vi "Live Capture Functional Stack.9.64bit.vi"() -> ()   [LabVIEW 2014]
uses:
  subvis/Stack Track.ctl
  subvis/Stack_State.ctl
  CameraControlTypeDef.ctl
  Desktop/camtiff/ctiff.llb/__CTIFFNewFileAndStyleUINT16.vi
  Desktop/camtiff/ctiff.llb/__CTIFFAddNewPageUINT16.vi
panel:
  in  "Preview":bool
  in  "Capture Mode":bool
  out "Record Ready":bool
  in  "Stacks":dbl=1.0
  in  "Time Lapse":bool
  out "Stack Frames":i32=100
  in  "Stack Frames":i32=100
  in  "Temp":path=path "C:/temp.tmp"
  in  "Frames":i32=100
  in  "HardDisk Record":bool
  in  "Internal Line Interval":dbl
  in  "Slit Width / Lines":sgl=150.0
  in  "Camera Readout Mode":u16(ring)=12 items=["Full Frame"=1, "Slit Scanning"=12]
  in  "Readout Direction":sgl(ring)=1.0 items=["Forward"=1, "Backward"=2]
  in  "Trigger Mode":sgl(ring)=1.0 items=["Normal"=1, "Start "=6]
  in  "Trigger Source":sgl(ring)=2.0 items=["Internal"=1, "External"=2]
  out "State":T1=enum."Start Sequence"
  out "Image":u16[][](graph)
  out "Saving":bool
  in  "AutoIncrement":bool=TRUE
  in  "Path":path=path "C:/Users/spim/Desktop/Craig Cap/temp/a.tiff"
  in  "Frames":i32=100
  out "Frame Index":i32
  out "error out":errorcluster
  in  "stop":bool
  in  "Ram Record":bool
  out "Total Frames":i32
  out "Elapsed Time":u32
  out "Software FPS":dbl
  out "Camera FPS":dbl
  in  "H Offset":i32 min=0 max=0 step=4
  in  "H Width":i32 min=4 max=2048 step=4
  out "SMD":dbl
  out "SHO":i32
  in  "V Offset":i32 min=0 max=0 step=4
  in  "V Width":i32 min=4 max=2048 step=4
  in  "Binning":u16(ring) items=["1x1"=1, "2x2"=2, "4x4"=4]
  out "SHW":i32
  out "SVO":i32
  out "SVW":i32
  in  "Scan Mode":dbl min=1.0 max=2.0 step=1.0
  in  "Exposure":dbl min=0.0010036691729323308 max=10.000004210526315 step=1e-08
  out "EXP":dbl
  out "Camera Model":string
  out "Camera Version":string
  out "Camera Serial":string
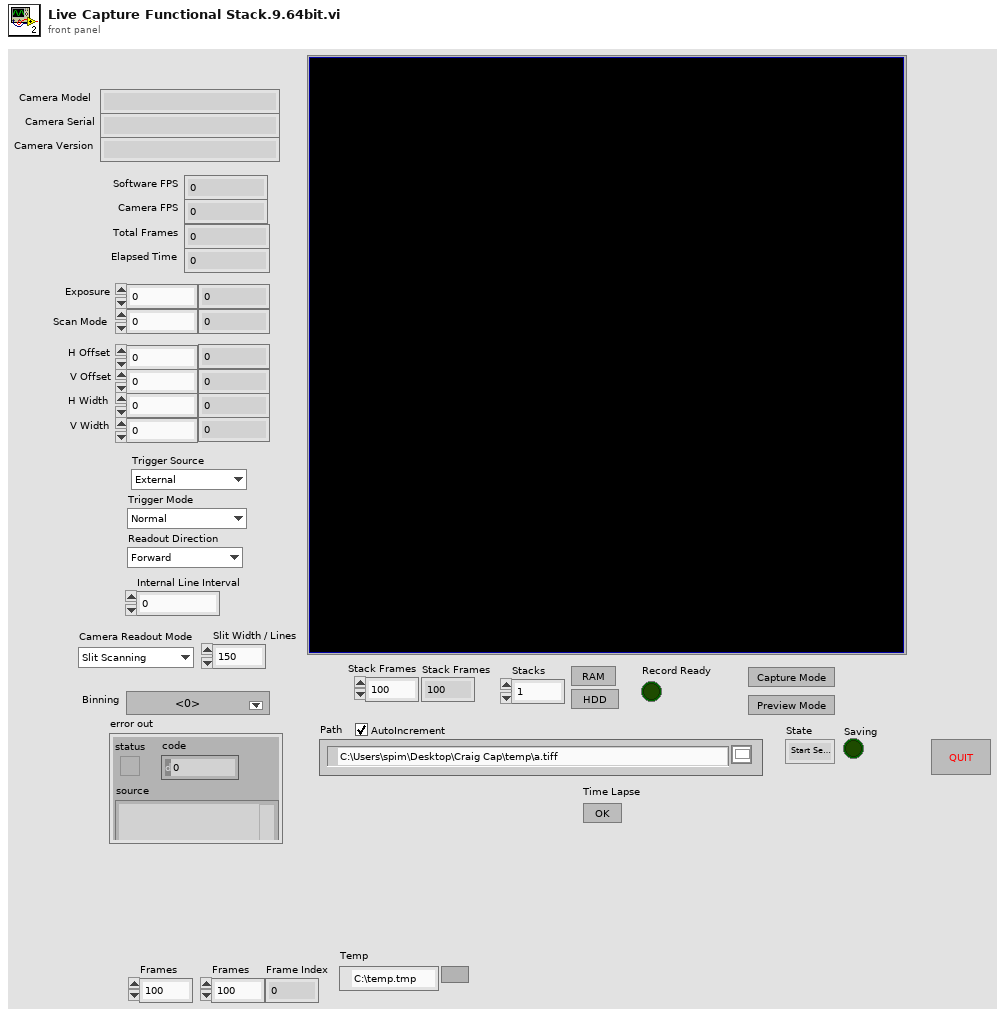
[diagram p1: front panel]
types:
  T1 = typedef "Stack Track.ctl" = enum16{"Idle", "Start Sequence", "Read Disk", "STOP", "Collecting", "End"}
  T2 = typedef "CameraControlTypeDef.ctl" = enum16{"IntervalLineInt", "Ram Record", "HardDisk Record", "Disengage Update", "Update", "Idle", "ROI", "Binning", "Scan Mode", "Trigger Mode", "Readout Mode", "Readout Direction", "Preview"}
  T3 = typedef "Stack_State.ctl" = cluster{"State":T1, "Stack Number":i32, "Image":u16[][]}
  T4 = enum8{"Enabled", "Disabled", "Disabled and Grayed Out"}
  T5 = cluster{"Model":string, "Camera ID":string, "Firmware":string}
  T6 = cluster{"Value":i32, "Minimum":i32, "Maximum":i32, "Increment":i32}
  T7 = cluster{"height":u32, "width":u32, "datatype":u32}
  T8 = cluster{"H Offset":i32, "V Offset":i32, "H Width":i32, "V Width":i32}
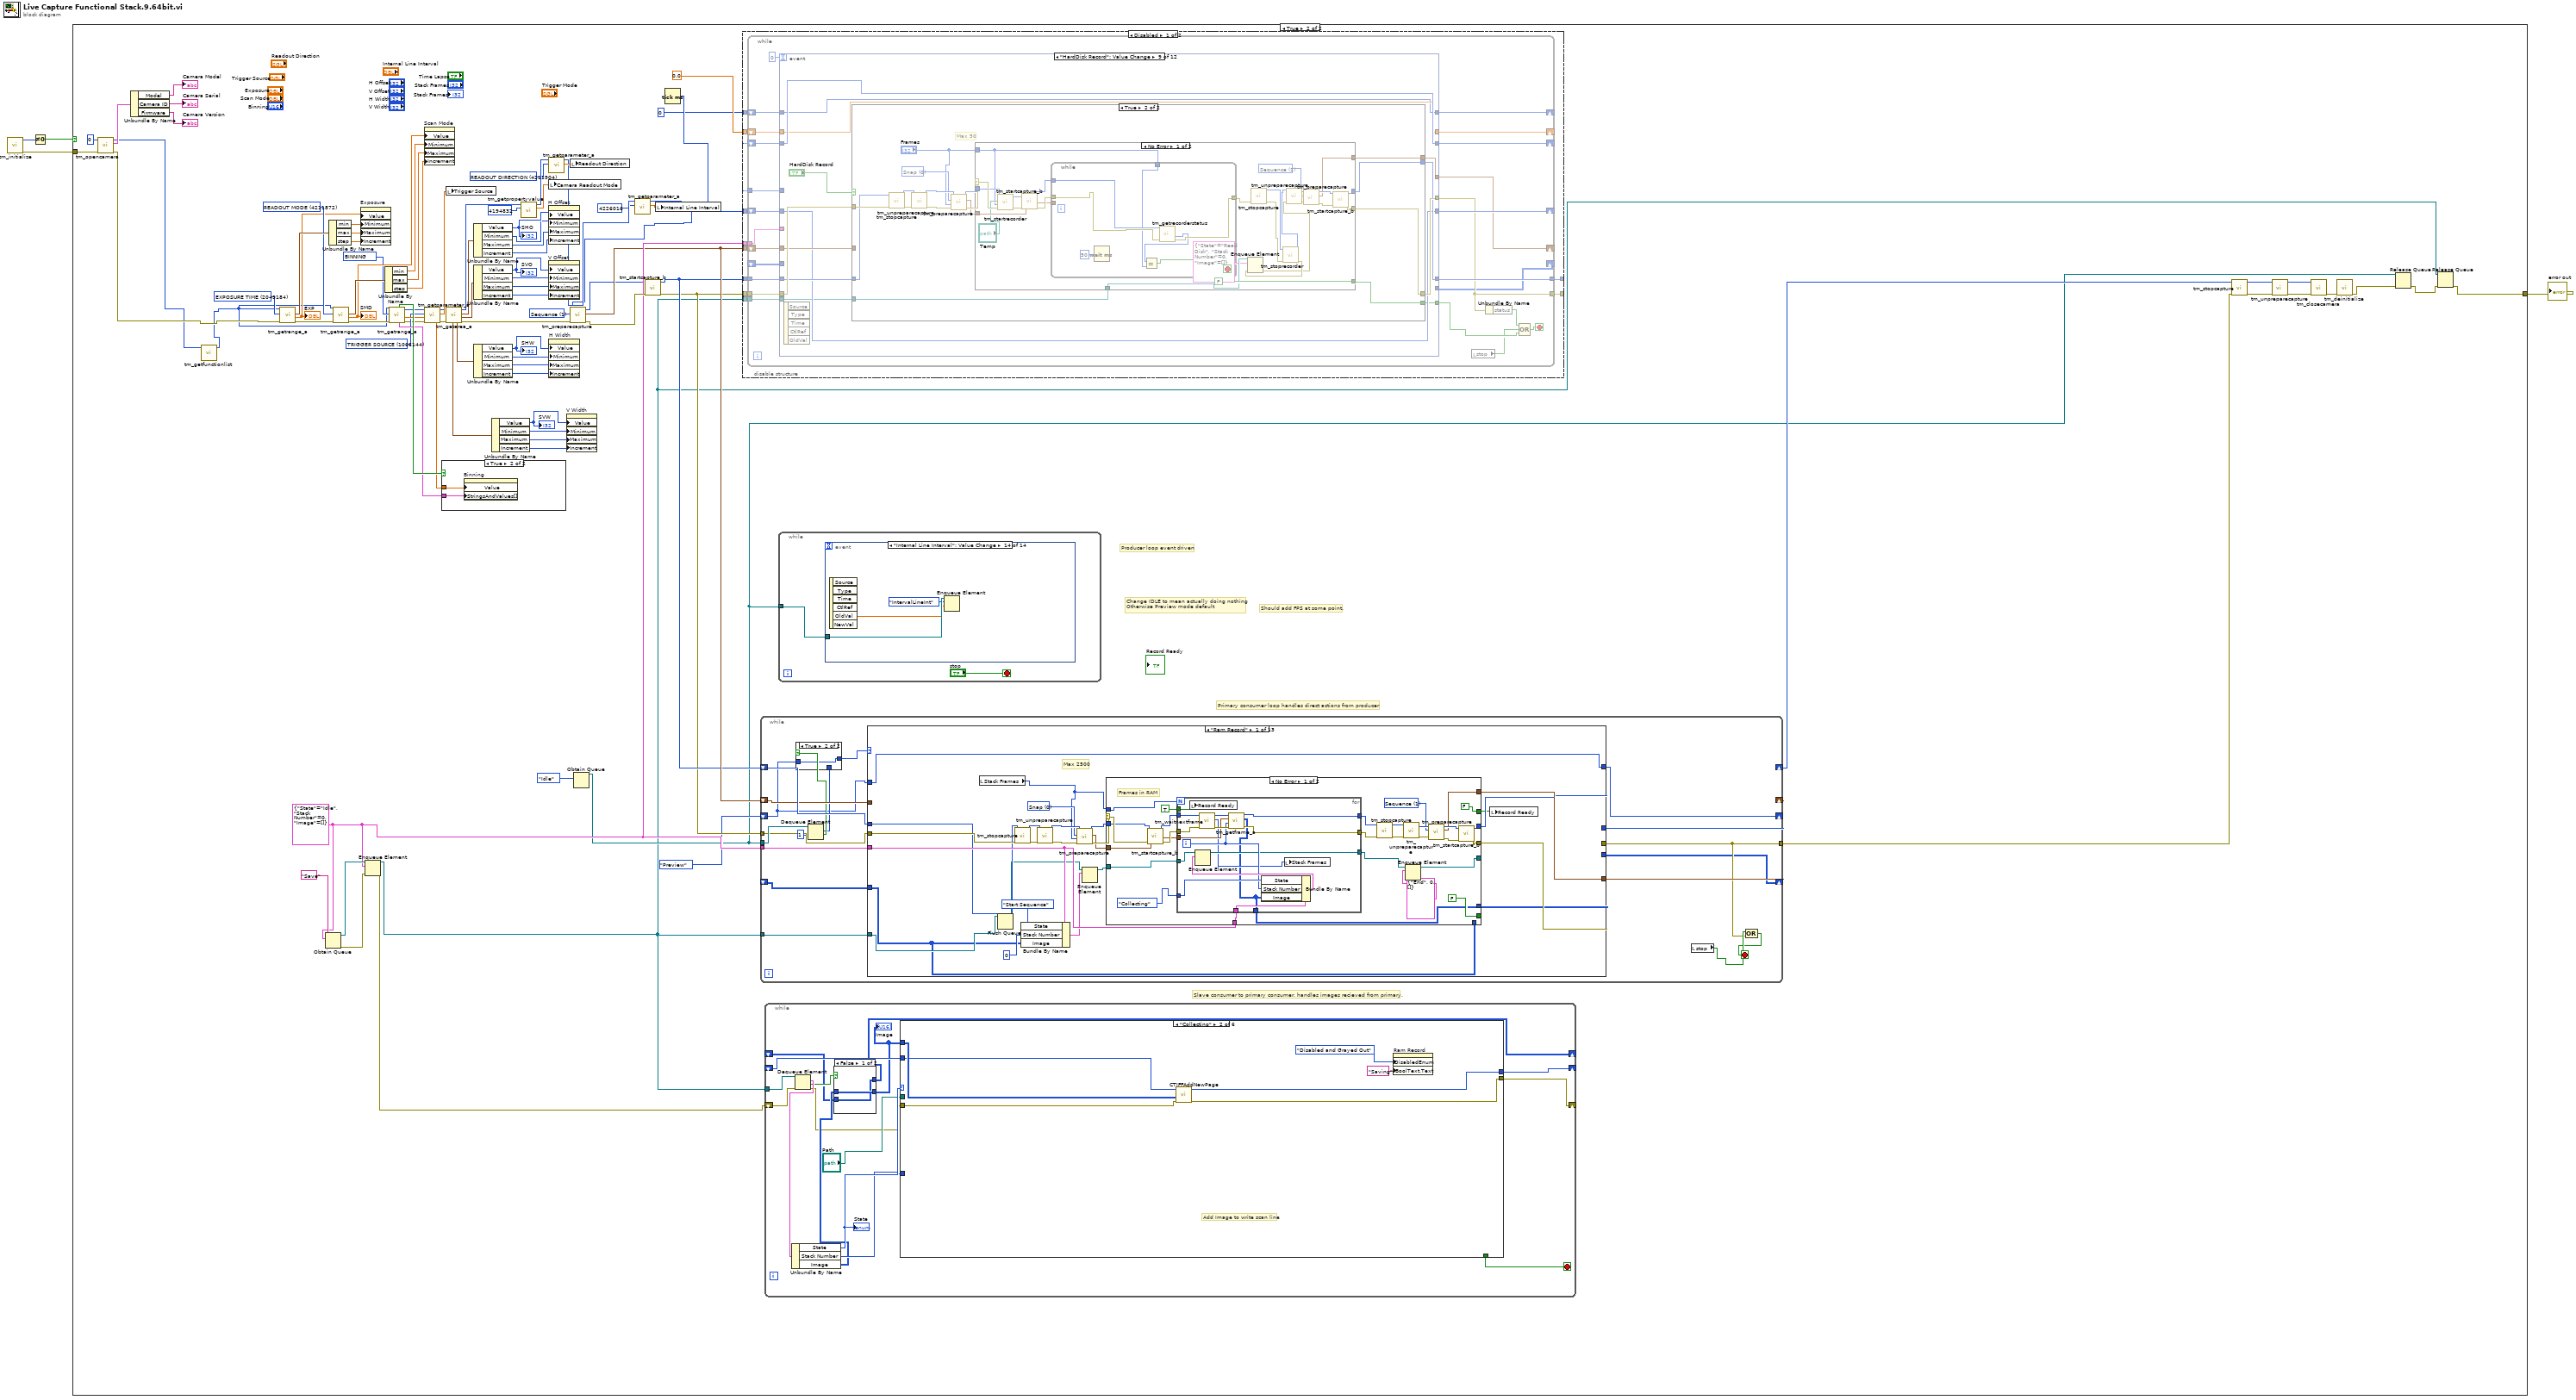
[diagram p0: block diagram]
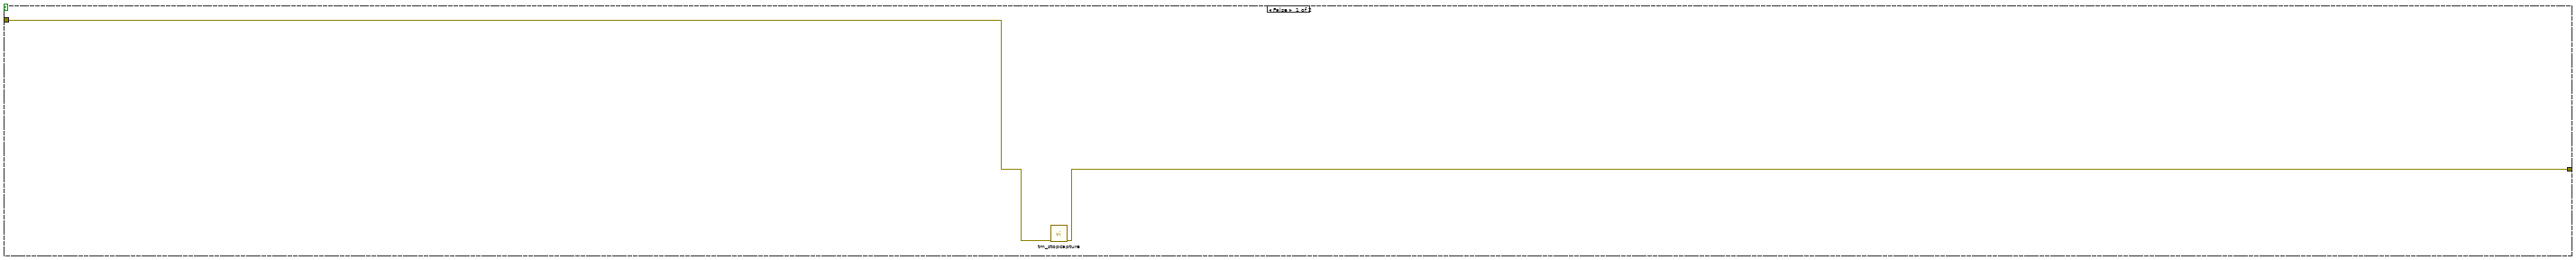
[diagram p2: hidden frame]
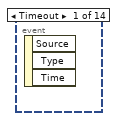
[diagram p3: hidden frame]
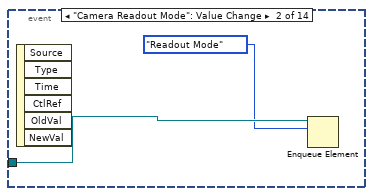
[diagram p4: hidden frame]
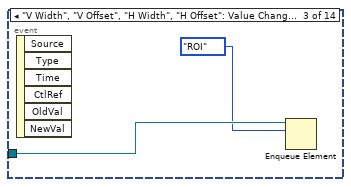
[diagram p5: hidden frame]
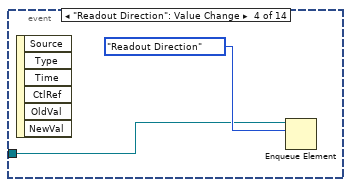
[diagram p6: hidden frame]
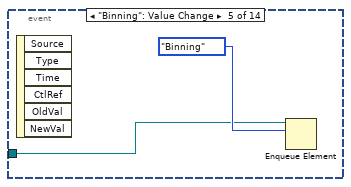
[diagram p7: hidden frame]
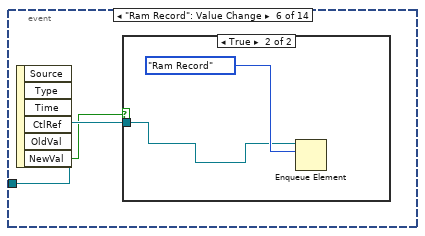
[diagram p8: hidden frame]
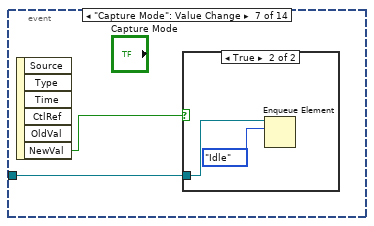
[diagram p10: hidden frame]
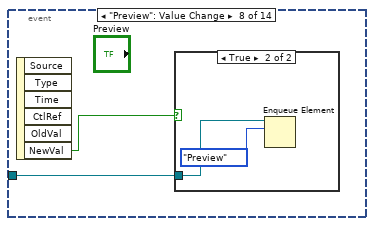
[diagram p12: hidden frame]
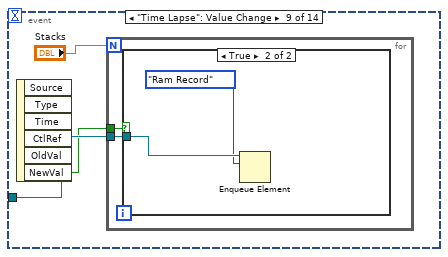
[diagram p14: hidden frame]
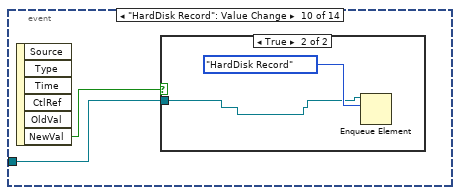
[diagram p16: hidden frame]
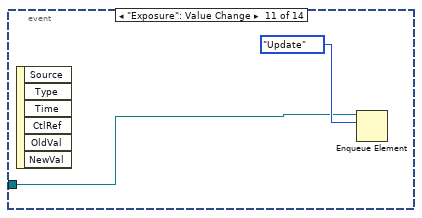
[diagram p18: hidden frame]
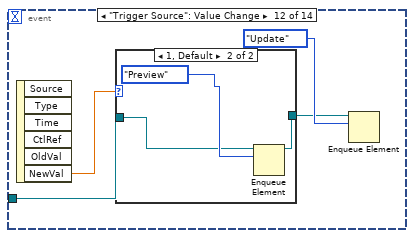
[diagram p19: hidden frame]
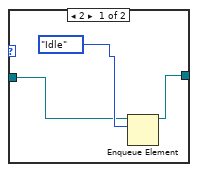
[diagram p20: hidden frame]
diagram:
  n1 = call <userlib>:"tm_initialize.vi"() -> ("error out"=w2:errorcluster, "Number Of Cameras"=w1:u32)  [unwired: 8 in, 2 out]
  n2 = Not Equal To 0?(x=w1) -> (x != 0?=w4:bool)
  n3 = case shown="True" w4 {
    tunnel: [w5 w15] -> w3
    tunnel: w2 -> [w6 w98]
    frame False {
      n4 = call <userlib>:"tm_stopcapture.vi"("error in (no error)"=w6) -> ("error out"=w5:errorcluster)  [unwired: 9 in, 1 out]
    }
    frame True {
      w33 = u32 4211904 items=["SENSOR MODE"=4212128, "CCD MODE"=4212384, "READOUT MODE"=4211872, "ACTIVE VIEW INDEX"=4343136, "BITS PER CHANNEL"=4342976, "IMAGE PIXEL TYPE"=4343296, "BINNING"=4215968, "EXPOSURE TIME"=2049184, "CONTRAST GAIN"=3163312, "CONTRAST OFFSET"=3163328, "LIGHT MODE"=2114720, "SENSITIVITY"=2114992, "PHOTON IMAGING MODE"=2115200, "HIGH DYNAMIC RANGE MODE"=3163360, "WHITE BALANCE"=3163568, "TEMPERATURE"=2115232, "TEMPERATURE TARGET"=2115264, "SENSOR COOLER FAN"=2115296, "LINEBUNDLE HEIGHT"=4212192, "MECHANICAL SHUTTER"=2115488, "BACK FOCUS POSITION"=8422304, "TRIGGER CONNECTOR"=1066432, "TRIGGER SOURCE"=1066144, "OUTPUT TRIGGER SOURCE"=1852576, "TRIGGER GLOBAL EXPOSURE"=2049680, "FIRST TRIGGER BEHAVIOR"=2049696, "CHANNEL SYNC"=1852352, "READOUT DIRECTION"=4211904, "PRE HSYNC COUNT"=1852704] ("Parameter")
      w42 = u32 1066144 items=["SENSOR MODE"=4212128, "CCD MODE"=4212384, "READOUT MODE"=4211872, "ACTIVE VIEW INDEX"=4343136, "BITS PER CHANNEL"=4342976, "IMAGE PIXEL TYPE"=4343296, "BINNING"=4215968, "EXPOSURE TIME"=2049184, "CONTRAST GAIN"=3163312, "CONTRAST OFFSET"=3163328, "LIGHT MODE"=2114720, "SENSITIVITY"=2114992, "PHOTON IMAGING MODE"=2115200, "HIGH DYNAMIC RANGE MODE"=3163360, "WHITE BALANCE"=3163568, "TEMPERATURE"=2115232, "TEMPERATURE TARGET"=2115264, "SENSOR COOLER FAN"=2115296, "LINEBUNDLE HEIGHT"=4212192, "MECHANICAL SHUTTER"=2115488, "BACK FOCUS POSITION"=8422304, "TRIGGER CONNECTOR"=1066432, "TRIGGER SOURCE"=1066144, "OUTPUT TRIGGER SOURCE"=1852576, "TRIGGER GLOBAL EXPOSURE"=2049680, "FIRST TRIGGER BEHAVIOR"=2049696, "CHANNEL SYNC"=1852352, "READOUT DIRECTION"=4211904, "PRE HSYNC COUNT"=1852704] ("Parameter")
      w28 = T3 {"State"=enum."Idle", "Stack Number"=0, "Image"=[]} ("input cluster")
      w47 = u32 2049184 items=["BINNING"=4215968, "BITS PER CHANNEL"=4342976, "ACTIVE VIEW INDEX"=4343136, "CCD MODE"=4212384, "SENSOR MODE"=4212128, "READOUT MODE"=4211872, "EXPOSURE TIME"=2049184, "CONTRAST GAIN"=3163312, "CONTRAST OFFSET"=3163328, "LIGHT MODE"=2114720, "SENSITIVITY"=2114992, "WHITE BALANCE"=3163568, "PHOTON IMAGING MODE"=2115200, "HIGH DYNAMIC RANGE MODE"=3163360, "TRIGGER SOURCE"=1066144, "TRIGGER ACTIVE"=1066160, "TRIGGER MODE"=1066400, "TRIGGER POLARITY"=1066416, "TRIGGER GLOBAL EXPOSURE"=2049680, "FIRST TRIGGER BEHAVIOR"=2049696, "TRIGGER TIMES"=1066448, "OUTPUT TRIGGER POLARITY"=1852592, "OUTPUT TRIGGER DELAY"=1852624, "OUTPUT TRIGGER PERIOD"=1852640, "TEMPERATURE"=2115232, "TEMPERATURE TARGET"=2115264, "SENSOR COOLER FAN"=2115296, "MECHANICAL SHUTTER"=2115488, "BACK FOCUS POSITION"=8422304, "FRAMEBUNDLE MODE"=4346784, "FRAMEBUNDLE NUMBER"=4346800, "LINEBUNDLE HEIGHT"=4212192, "TRIGGER CONNECTOR"=1066432, "IMAGE PIXEL TYPE"=4343296, "OUTPUT TRIGGER KIND"=1852656, "READOUT DIRECTION"=4211904, "CHANNEL SYNC"=1852352] ("Parameter")
      w48 = u32 4211872 items=["BINNING"=4215968, "BITS PER CHANNEL"=4342976, "ACTIVE VIEW INDEX"=4343136, "CCD MODE"=4212384, "SENSOR MODE"=4212128, "READOUT MODE"=4211872, "EXPOSURE TIME"=2049184, "CONTRAST GAIN"=3163312, "CONTRAST OFFSET"=3163328, "LIGHT MODE"=2114720, "SENSITIVITY"=2114992, "WHITE BALANCE"=3163568, "PHOTON IMAGING MODE"=2115200, "HIGH DYNAMIC RANGE MODE"=3163360, "TRIGGER SOURCE"=1066144, "TRIGGER ACTIVE"=1066160, "TRIGGER MODE"=1066400, "TRIGGER POLARITY"=1066416, "TRIGGER GLOBAL EXPOSURE"=2049680, "FIRST TRIGGER BEHAVIOR"=2049696, "TRIGGER TIMES"=1066448, "OUTPUT TRIGGER POLARITY"=1852592, "OUTPUT TRIGGER DELAY"=1852624, "OUTPUT TRIGGER PERIOD"=1852640, "TEMPERATURE"=2115232, "TEMPERATURE TARGET"=2115264, "SENSOR COOLER FAN"=2115296, "MECHANICAL SHUTTER"=2115488, "BACK FOCUS POSITION"=8422304, "FRAMEBUNDLE MODE"=4346784, "FRAMEBUNDLE NUMBER"=4346800, "LINEBUNDLE HEIGHT"=4212192, "TRIGGER CONNECTOR"=1066432, "IMAGE PIXEL TYPE"=4343296, "OUTPUT TRIGGER KIND"=1852656, "READOUT DIRECTION"=4211904, "CHANNEL SYNC"=1852352] ("Parameter")
      w49 = u32 4215968 items=["BINNING"=4215968, "BITS PER CHANNEL"=4342976, "ACTIVE VIEW INDEX"=4343136, "CCD MODE"=4212384, "SENSOR MODE"=4212128, "READOUT MODE"=4211872, "EXPOSURE TIME"=2049184, "CONTRAST GAIN"=3163312, "CONTRAST OFFSET"=3163328, "LIGHT MODE"=2114720, "SENSITIVITY"=2114992, "WHITE BALANCE"=3163568, "PHOTON IMAGING MODE"=2115200, "HIGH DYNAMIC RANGE MODE"=3163360, "TRIGGER SOURCE"=1066144, "TRIGGER ACTIVE"=1066160, "TRIGGER MODE"=1066400, "TRIGGER POLARITY"=1066416, "TRIGGER GLOBAL EXPOSURE"=2049680, "FIRST TRIGGER BEHAVIOR"=2049696, "TRIGGER TIMES"=1066448, "OUTPUT TRIGGER POLARITY"=1852592, "OUTPUT TRIGGER DELAY"=1852624, "OUTPUT TRIGGER PERIOD"=1852640, "TEMPERATURE"=2115232, "TEMPERATURE TARGET"=2115264, "SENSOR COOLER FAN"=2115296, "MECHANICAL SHUTTER"=2115488, "BACK FOCUS POSITION"=8422304, "FRAMEBUNDLE MODE"=4346784, "FRAMEBUNDLE NUMBER"=4346800, "LINEBUNDLE HEIGHT"=4212192, "TRIGGER CONNECTOR"=1066432, "IMAGE PIXEL TYPE"=4343296, "OUTPUT TRIGGER KIND"=1852656, "READOUT DIRECTION"=4211904, "CHANNEL SYNC"=1852352] ("Parameter")
      w94 = 1 items=["Snap", "Sequence"] ("Capture mode")
      # "Change IDLE to mean actually doing nothing\nOtherwise Preview mode default"
      # "Slave consumer to primary consumer, handles images recieved from primary."
      # "Primary consumer loop handles direct actions from producer"
      # "Producer loop event driven"
      # "Should add FPS at some point."
      n5 = call <userlib>:"tm_opencamera.vi"("error in (no error)"=w98, "Camera Index"=u32 0) -> ("error out"=w29:errorcluster, "Camera Details"=w61:T5, "Handle out"=w13:u32)  [unwired: 7 in]
      n6 = Unbundle By Name(w61) -> ("Model"=→"Camera Model":string, "Camera ID"=→"Camera Serial":string, "Firmware"=→"Camera Version":string)
      n7 = call <userlib>:"tm_getfunctionlist.vi"("Handle in"=w13) -> ("Handle out"=w12:u32)  [unwired: 8 in, 2 out]
      n8 = call <userlib>:"tm_getrange_a.vi"("error in (no error)"=w29, "Parameter"=w47, "Handle in"=w12) -> ("error out"=w56:errorcluster, "default"=w45:dbl, "Range"=w57:cluster{"min":dbl, "max":dbl, "step":dbl})  [unwired: 2 in, 4 out]
      "EXP" <- w45
      n9 = Obtain Queue(name (unnamed)="Save", element data type=w28) -> (queue out=w31:refnum<queue>, error out=w10:errorcluster)  [unwired: 3 in, 1 out]
      n10 = Unbundle By Name(w57) -> ("min"=w92:dbl, "max"=w91:dbl, "step"=w90:dbl)
      n11 = call <userlib>:"tm_getrange_a.vi"("error in (no error)"=w56, "Parameter"=w48, "Handle in"=w12) -> ("error out"=w53:errorcluster, "default"=w54:dbl, "Range"=w55:cluster{"min":dbl, "max":dbl, "step":dbl})  [unwired: 2 in, 4 out]
      "SMD" <- w54
      n12 = property on="Exposure" class="DigNum (strict)"("Value"=w45, "Minimum"=w92, "Maximum"=w91, "Increment"=w90) -> ()  [unwired: 2 in, 2 out]
      n13 = Enqueue Element(queue=w31, element=w28, error in (no error)=w10) -> (queue out=w14:refnum<queue>, error out=w9:errorcluster)  [unwired: 1 in, 1 out]
      n14 = Unbundle By Name(w55) -> ("min"=w89:dbl, "max"=w88:dbl, "step"=w87:dbl)
      n15 = call <userlib>:"tm_getrange_a.vi"("error in (no error)"=w53, "Parameter"=w49, "Handle in"=w12) -> ("error out"=w39:errorcluster, "default"=w51:dbl, "Handle out"=w41:u32, "Value Names"=w50:cluster{"Name":string, "Value":dbl}[], "Writable"=w52:bool)  [unwired: 2 in, 2 out]
      n16 = property on="Scan Mode" class="DigNum (strict)"("Value"=w54, "Minimum"=w89, "Maximum"=w88, "Increment"=w87) -> ()  [unwired: 2 in, 2 out]
      n17 = call <userlib>:"tm_getparameter_a.vi"("error in (no error)"=w39, "Parameter"=w42, "Handle in"=w41) -> ("error out"=w38:errorcluster, "Value out"=w43:dbl, "Handle out"=w40:u32)  [unwired: 6 in]
      n18 = case shown="True" w52 {
        tunnel: w50 -> [_ w1177]
        tunnel: w51 -> [_ w1176]
        frame False {
        }
        frame True {
          n19 = property on="Binning" class="Ring (strict)"("Value"=w1176, "StringsAndValues[]"=w1177) -> ()  [unwired: 2 in, 2 out]
        }
      }
      n20 = local write "Trigger Source"(w43) -> ()
      n21 = call <userlib>:"tm_getarea_a.vi"("error in (no error)"=w38, "Handle in"=w40) -> ("error out"=w44:errorcluster, "V Offset"=w86:T6, "H Offset"=w67:T6, "Handle out"=w35:u32, "H Width"=w85:T6, "V Width"=w84:T6)  [unwired: 4 in]
      n22 = Unbundle By Name(w67) -> ("Value"=w66:i32, "Minimum"=w65:i32, "Maximum"=w64:i32, "Increment"=w63:i32)
      "SHO" <- w66
      n23 = Unbundle By Name(w86) -> ("Value"=w74:i32, "Minimum"=w83:i32, "Maximum"=w82:i32, "Increment"=w81:i32)
      "SVO" <- w74
      n24 = Unbundle By Name(w85) -> ("Value"=w73:i32, "Minimum"=w80:i32, "Maximum"=w79:i32, "Increment"=w78:i32)
      "SHW" <- w73
      n25 = Unbundle By Name(w84) -> ("Value"=w72:i32, "Minimum"=w77:i32, "Maximum"=w76:i32, "Increment"=w75:i32)
      "SVW" <- w72
      n26 = call <userlib>:"tm_getpropertyvalue.vi"("Property ID"=u32 4194832, "Handle in"=w35) -> ("Value in"=w36:sgl, "Handle out"=w34:u32)  [unwired: 7 in, 1 out]
      n27 = call <userlib>:"tm_getparameter_a.vi"("Parameter"=w33, "Handle in"=w34) -> ("Value out"=w32:dbl, "Handle out"=w19:u32)  [unwired: 7 in, 1 out]
      n28 = local write "Camera Readout Mode"(w36) -> ()
      n29 = property on="H Offset" class="DigNum (strict)"("Value"=w66, "Minimum"=w65, "Maximum"=w64, "Increment"=w63) -> ()  [unwired: 2 in, 2 out]
      n30 = property on="V Offset" class="DigNum (strict)"("Value"=w74, "Minimum"=w83, "Maximum"=w82, "Increment"=w81) -> ()  [unwired: 2 in, 2 out]
      n31 = property on="H Width" class="DigNum (strict)"("Value"=w73, "Minimum"=w80, "Maximum"=w79, "Increment"=w78) -> ()  [unwired: 2 in, 2 out]
      n32 = property on="V Width" class="DigNum (strict)"("Value"=w72, "Minimum"=w77, "Maximum"=w76, "Increment"=w75) -> ()  [unwired: 2 in, 2 out]
      n33 = local write "Readout Direction"(w32) -> ()
      n34 = Obtain Queue(element data type=CameraControlTypeDef."Idle" ("Enum")) -> (queue out=w17:refnum<queue>)  [unwired: 4 in, 2 out]
      n35 = call <userlib>:"tm_getparameter_a.vi"("Parameter"=4226016, "Handle in"=w19) -> ("Value out"=w7:dbl, "Handle out"=w8:u32)  [unwired: 7 in, 1 out]
      n36 = call <userlib>:"tm_preparecapture.vi"("error in (no error)"=w44, "Capture mode"=w94, "Handle in"=w8) -> ("error out"=w30:errorcluster, "Buffer Info"=w27:T7, "Handle out"=w20:u32)  [unwired: 5 in, 1 out]
      n37 = call <userlib>:"tm_startcapture_b.vi"("error in (no error)"=w30, "Handle in"=w20) -> ("error out"=w25:errorcluster, "Handle out"=w26:u32)  [unwired: 8 in]
      n38 = local write "Internal Line Interval"(w7) -> ()
      n39 = Tick Count (ms)() -> (millisecond timer value=w93:u32)
      n40 = disable-structure shown="Disabled" {
        disable-tunnel: 0.0 -> [w592 _]
        disable-tunnel: w93 -> [w591 _]
        disable-tunnel: 0 -> [w590 _]
        disable-tunnel: [w589 _] -> _
        disable-tunnel: [w588 _] -> _
        disable-tunnel: w28 -> [w587 _]
        disable-tunnel: w27 -> [w586 _]
        disable-tunnel: w26 -> [w585 _]
        disable-tunnel: w25 -> [w584 _]
        disable-tunnel: w14 -> [w583 _]
        frame Disabled {
          n41 = while {
            tunnel: w584 -> [w606]
            tunnel: [w604] -> w588
            tunnel: [w603] -> w589
            shift-right: [w613] -> _
            shift-left: w591 -> [w611]
            shift-right: [w614] -> _
            shift-left: w592 -> [w612]
            shift-right: [w605] -> _
            shift-left: w591 -> [w609]
            tunnel: w585 -> [w607]
            tunnel: w591 -> [w610]
            shift-right: [w602] -> _
            shift-left: w586 -> [w608]
            shift-right: [w600] -> _
            shift-left: w590 -> [w601]
            tunnel: w583 -> [w599]
            shift-right: [w597] -> _
            shift-left: _ -> [w596]
            tunnel: w587 -> [w595]
            stop <- w615 stop-if-true
            n42 = event shown="[8] \"HardDisk Record\": Value Change" {
              selector: _ -> [_ _ _ _ _ _ _ _ _ _ _ _]
              dyn-events: _ -> [_ _ _ _ _ _ _ _ _ _ _ _]
              timeout: 0 -> [_ _ _ _ _ _ _ _ _ _ _ _]
              tunnel: [w626 w695 w709 w722 w741 w761 w783 w811 w908 w1002 w1038 w1083] -> w614
              tunnel: [w625 w696 w710 w723 w742 w762 w784 w812 w909 w1003 w1039 w1084] -> w613
              tunnel: w612 -> [w637 w695 w709 w722 w741 w761 w783 w811 w908 w1002 w1038 w1083]
              tunnel: w611 -> [w628 w696 w710 w723 w742 w762 w784 w812 w909 w1003 w1039 w1084]
              tunnel: w610 -> [w633 _ _ _ _ _ _ _ _ _ _ _]
              tunnel: w609 -> [w638 w697 w711 w724 w743 w763 w785 w807 w904 w1004 w1046 w1091]
              tunnel: w608 -> [w632 w694 w708 w721 _ w760 _ w808 w905 _ _ _]
              tunnel: w607 -> [w640 w690 w703 w717 w736 w754 w776 w815 w912 w999 w1015 w1053]
              tunnel: w606 -> [w639 w692 w699 w718 w735 w757 w775 w816 w913 w998 w1014 w1052]
              tunnel: [w636 w697 w711 w724 w743 w763 w785 w807 w904 w1004 w1046 w1091] -> w605
              tunnel: [w635 w687 w706 w714 w727 w747 w766 w813 w910 w993 w1041 w1086] -> w604
              tunnel: [w634 w686 w705 w713 w726 w746 w764 w814 w911 w994 w1042 w1087] -> w603
              tunnel: [w631 w694 w708 w721 w730 w760 w771 w809 w906 w992 w1040 w1085] -> w602
              tunnel: w601 -> [w623 w693 w707 w720 w740 w759 w782 w810 w907 w991 w1011 w1047]
              tunnel: [w622 w693 w707 w720 w740 w759 w782 w810 w907 w991 w1011 w1047] -> w600
              tunnel: w599 -> [w617 _ _ _ _ _ _ w806 w903 _ _ _]
              tunnel: [_ _ _ _ _ _ _ w805 w902 _ _ _] -> w598
              tunnel: w595 -> [w620 _ _ _ _ _ _ w803 _ _ _ _]
              tunnel: [w619 _ _ _ _ _ _ _ _ _ _ _] -> w597
              tunnel: w596 -> [w618 _ _ _ _ _ _ w804 _ _ _ _]
              event Timeout {
                n43 = event-data() -> ()  [unwired: 1 in, 2 out]
                n44 = call <userlib>:"tm_waitnextframe.vi"("error in (no error)"=w639, "Handle in"=w640) -> ("error out"=w643:errorcluster, "Frame Count"=w624:i32, "Frame Index"=w642:i32, "Handle out"=w644:u32)  [unwired: 6 in]
                "Total Frames" <- w624
                n45 = Tick Count (ms)() -> (millisecond timer value=w630:u32)
                n46 = Increment(x=w637) -> (x+1=w627:dbl)
                n47 = Subtract(x=w630, y=w633) -> (x-y=→"Elapsed Time":u32)
                n48 = Add(x=w628, y=u32 1000) -> (x+y=w648:u32)
                n49 = Less Or Equal?(x=w648, y=w630) -> (x <= y?=w629:bool)
                n50 = Add(x=w638, y=u32 50) -> (x+y=w646:u32)
                n51 = Less Or Equal?(x=w646, y=w630) -> (x <= y?=w621:bool)
                n52 = case shown="True" w629 {
                  tunnel: w628 -> [w651 w660]
                  tunnel: [w651 w657] -> w625
                  tunnel: w627 -> [w650 w663]
                  tunnel: w630 -> [_ w657]
                  tunnel: [w650 0.0] -> w626
                  tunnel: w624 -> [_ w652]
                  tunnel: w623 -> [w649 w655]
                  tunnel: [w649 w652] -> w622
                  frame False {
                  }
                  frame True {
                    n53 = Subtract(x=w657, y=w660) -> (x-y=w659:u32)
                    n54 = Subtract(x=w652, y=w655) -> (x-y=w653:i32)
                    n55 = To Double Precision Float(number=w659) -> (double precision float=w665:dbl)
                    n56 = Divide(x=w665, y=1000.0) -> (x/y=w656:dbl)
                    n57 = To Double Precision Float(number=w653) -> (double precision float=w654:dbl)
                    n58 = Divide(x=w654, y=w656) -> (x/y=→"Camera FPS":dbl)
                    n59 = Divide(x=w663, y=w656) -> (x/y=→"Software FPS":dbl)
                  }
                }
                n60 = case shown="True" w621 {
                  tunnel: w638 -> [w670 _]
                  tunnel: w630 -> [_ w683]
                  tunnel: [w670 w683] -> w636
                  tunnel: w644 -> [w669 w682]
                  tunnel: w632 -> [w667 w677]
                  tunnel: w643 -> [w668 w681]
                  tunnel: [w669 w680] -> w635
                  tunnel: [w668 w679] -> w634
                  tunnel: w642 -> [_ w678]
                  tunnel: [w667 w677] -> w631
                  tunnel: w617 -> [_ w676]
                  tunnel: w620 -> [_ w672]
                  tunnel: [w666 w671] -> w619
                  tunnel: w618 -> [w666 _]
                  frame False {
                  }
                  frame True {
                    n61 = call <userlib>:"tm_getframe_a.vi"("error in (no error)"=w681, "Frame Index"=w678, "Buffer Info"=w677, "Handle in"=w682) -> ("error out"=w679:errorcluster, "Data 16"=w671:u16[][], "Handle out"=w680:u32)  [unwired: 3 in, 2 out]
                    n62 = Bundle By Name(cluster=w672, "State"=Stack_Track."Idle", "Stack Number"=0, "Image"=w671) -> (w673:T3)
                    n63 = Enqueue Element(queue=w676, element=w673) -> ()  [unwired: 2 in, 3 out]
                  }
                }
              }
              event "Exposure": Value Change {
                w685 = u32 2049184 items=["SENSOR MODE"=4212128, "CCD MODE"=4212384, "READOUT MODE"=4211872, "ACTIVE VIEW INDEX"=4343136, "BITS PER CHANNEL"=4342976, "IMAGE PIXEL TYPE"=4343296, "BINNING"=4215968, "EXPOSURE TIME"=2049184, "CONTRAST GAIN"=3163312, "CONTRAST OFFSET"=3163328, "LIGHT MODE"=2114720, "SENSITIVITY"=2114992, "PHOTON IMAGING MODE"=2115200, "HIGH DYNAMIC RANGE MODE"=3163360, "WHITE BALANCE"=3163568, "TEMPERATURE"=2115232, "TEMPERATURE TARGET"=2115264, "SENSOR COOLER FAN"=2115296, "LINEBUNDLE HEIGHT"=4212192, "MECHANICAL SHUTTER"=2115488, "BACK FOCUS POSITION"=8422304, "TRIGGER CONNECTOR"=1066432, "TRIGGER SOURCE"=1066144, "OUTPUT TRIGGER SOURCE"=1852576, "TRIGGER GLOBAL EXPOSURE"=2049680, "FIRST TRIGGER BEHAVIOR"=2049696, "CHANNEL SYNC"=1852352, "READOUT DIRECTION"=4211904, "PRE HSYNC COUNT"=1852704] ("Parameter")
                n64 = event-data() -> ("NewVal"=w691:dbl)  [unwired: 1 in, 2 out]
                n65 = call <userlib>:"tm_setparameter_a.vi"("error in (no error)"=w692, "Value in"=w691, "Parameter"=w685, "Handle in"=w690) -> ("error out"=w689:errorcluster, "Handle out"=w688:u32)  [unwired: 6 in]
                n66 = call <userlib>:"tm_getparameter_a.vi"("error in (no error)"=w689, "Parameter"=w685, "Handle in"=w688) -> ("error out"=w686:errorcluster, "Value out"=w684:dbl, "Handle out"=w687:u32)  [unwired: 6 in]
                n67 = local write "EXP"(w684) -> ()
              }
              event "Internal Line Interval": Value Change {
                w698 = u32 4191424 items=["SENSOR MODE"=4212128, "CCD MODE"=4212384, "READOUT MODE"=4211872, "ACTIVE VIEW INDEX"=4343136, "BITS PER CHANNEL"=4342976, "IMAGE PIXEL TYPE"=4343296, "BINNING"=4215968, "EXPOSURE TIME"=2049184, "CONTRAST GAIN"=3163312, "CONTRAST OFFSET"=3163328, "LIGHT MODE"=2114720, "SENSITIVITY"=2114992, "PHOTON IMAGING MODE"=2115200, "HIGH DYNAMIC RANGE MODE"=3163360, "WHITE BALANCE"=3163568, "TEMPERATURE"=2115232, "TEMPERATURE TARGET"=2115264, "SENSOR COOLER FAN"=2115296, "LINEBUNDLE HEIGHT"=4212192, "MECHANICAL SHUTTER"=2115488, "BACK FOCUS POSITION"=8422304, "TRIGGER CONNECTOR"=1066432, "TRIGGER SOURCE"=1066144, "OUTPUT TRIGGER SOURCE"=1852576, "TRIGGER GLOBAL EXPOSURE"=2049680, "FIRST TRIGGER BEHAVIOR"=2049696, "CHANNEL SYNC"=1852352, "READOUT DIRECTION"=4211904, "PRE HSYNC COUNT"=1852704, "INTERNAL LINE SPEED"=4191408, "INTERNAL LINE INVERVAL"=4191424] ("Parameter")
                n68 = event-data() -> ("NewVal"=w702:dbl)  [unwired: 1 in, 2 out]
                n69 = call <userlib>:"tm_setparameter_a.vi"("error in (no error)"=w699, "Value in"=w702, "Parameter"=w698, "Handle in"=w703) -> ("error out"=w700:errorcluster, "Handle out"=w701:u32)  [unwired: 6 in]
                n70 = call <userlib>:"tm_getparameter_a.vi"("error in (no error)"=w700, "Parameter"=w698, "Handle in"=w701) -> ("error out"=w705:errorcluster, "Value out"=w704:dbl, "Handle out"=w706:u32)  [unwired: 6 in]
                n71 = local write "Internal Line Interval"(w704) -> ()
              }
              event "Trigger Source": Value Change {
                w719 = u32 1066144 items=["SENSOR MODE"=4212128, "CCD MODE"=4212384, "READOUT MODE"=4211872, "ACTIVE VIEW INDEX"=4343136, "BITS PER CHANNEL"=4342976, "IMAGE PIXEL TYPE"=4343296, "BINNING"=4215968, "EXPOSURE TIME"=2049184, "CONTRAST GAIN"=3163312, "CONTRAST OFFSET"=3163328, "LIGHT MODE"=2114720, "SENSITIVITY"=2114992, "PHOTON IMAGING MODE"=2115200, "HIGH DYNAMIC RANGE MODE"=3163360, "WHITE BALANCE"=3163568, "TEMPERATURE"=2115232, "TEMPERATURE TARGET"=2115264, "SENSOR COOLER FAN"=2115296, "LINEBUNDLE HEIGHT"=4212192, "MECHANICAL SHUTTER"=2115488, "BACK FOCUS POSITION"=8422304, "TRIGGER CONNECTOR"=1066432, "TRIGGER SOURCE"=1066144, "OUTPUT TRIGGER SOURCE"=1852576, "TRIGGER GLOBAL EXPOSURE"=2049680, "FIRST TRIGGER BEHAVIOR"=2049696, "CHANNEL SYNC"=1852352, "READOUT DIRECTION"=4211904, "PRE HSYNC COUNT"=1852704] ("Parameter")
                n72 = event-data() -> ("NewVal"=w712:sgl)  [unwired: 1 in, 3 out]
                n73 = call <userlib>:"tm_setparameter_a.vi"("error in (no error)"=w718, "Value in"=w712, "Parameter"=w719, "Handle in"=w717) -> ("error out"=w716:errorcluster, "Handle out"=w715:u32)  [unwired: 6 in]
                n74 = call <userlib>:"tm_getparameter_a.vi"("error in (no error)"=w716, "Parameter"=w719, "Handle in"=w715) -> ("error out"=w713:errorcluster, "Handle out"=w714:u32)  [unwired: 6 in, 1 out]
              }
              event "Trigger Mode": Value Change {
                w731 = 1 items=["Snap", "Sequence"] ("Capture mode")
                n75 = event-data() -> ("NewVal"=w725:sgl)  [unwired: 1 in, 4 out]
                n76 = call <userlib>:"tm_stopcapture.vi"("error in (no error)"=w735, "Handle in"=w736) -> ("error out"=w738:errorcluster, "Handle out"=w737:u32)  [unwired: 8 in]
                n77 = call <userlib>:"tm_unpreparecapture.vi"("error in (no error)"=w738, "Handle in"=w737) -> ("error out"=w734:errorcluster, "Handle out"=w733:u32)  [unwired: 8 in]
                n78 = call <userlib>:"tm_setpropertyvalue.vi"("error in (no error)"=w734, "Value in"=w725, "Property ID"=u32 1049104, "Handle in"=w733) -> ("error out"=w729:errorcluster, "Handle out"=w732:u32)  [unwired: 6 in]
                n79 = call <userlib>:"tm_preparecapture.vi"("Capture mode"=w731, "Handle in"=w732) -> ("Buffer Info"=w730:T7, "Handle out"=w728:u32)  [unwired: 6 in, 2 out]
                n80 = call <userlib>:"tm_startcapture_b.vi"("error in (no error)"=w729, "Handle in"=w728) -> ("error out"=w726:errorcluster, "Handle out"=w727:u32)  [unwired: 8 in]
              }
              event "Readout Direction": Value Change {
                w752 = 1 items=["Snap", "Sequence"] ("Capture mode")
                w745 = u32 4211904 items=["SENSOR MODE"=4212128, "CCD MODE"=4212384, "READOUT MODE"=4211872, "ACTIVE VIEW INDEX"=4343136, "BITS PER CHANNEL"=4342976, "IMAGE PIXEL TYPE"=4343296, "BINNING"=4215968, "EXPOSURE TIME"=2049184, "CONTRAST GAIN"=3163312, "CONTRAST OFFSET"=3163328, "LIGHT MODE"=2114720, "SENSITIVITY"=2114992, "PHOTON IMAGING MODE"=2115200, "HIGH DYNAMIC RANGE MODE"=3163360, "WHITE BALANCE"=3163568, "TEMPERATURE"=2115232, "TEMPERATURE TARGET"=2115264, "SENSOR COOLER FAN"=2115296, "LINEBUNDLE HEIGHT"=4212192, "MECHANICAL SHUTTER"=2115488, "BACK FOCUS POSITION"=8422304, "TRIGGER CONNECTOR"=1066432, "TRIGGER SOURCE"=1066144, "OUTPUT TRIGGER SOURCE"=1852576, "TRIGGER GLOBAL EXPOSURE"=2049680, "FIRST TRIGGER BEHAVIOR"=2049696, "CHANNEL SYNC"=1852352, "READOUT DIRECTION"=4211904, "PRE HSYNC COUNT"=1852704] ("Parameter")
                n81 = event-data() -> ("NewVal"=w744:sgl)  [unwired: 1 in, 3 out]
                n82 = call <userlib>:"tm_stopcapture.vi"("error in (no error)"=w757, "Handle in"=w754) -> ("error out"=w758:errorcluster, "Handle out"=w753:u32)  [unwired: 8 in]
                n83 = call <userlib>:"tm_unpreparecapture.vi"("error in (no error)"=w758, "Handle in"=w753) -> ("error out"=w756:errorcluster, "Handle out"=w755:u32)  [unwired: 8 in]
                n84 = call <userlib>:"tm_setparameter_a.vi"("error in (no error)"=w756, "Value in"=w744, "Parameter"=w745, "Handle in"=w755) -> ("error out"=w749:errorcluster, "Handle out"=w748:u32)  [unwired: 6 in]
                n85 = call <userlib>:"tm_preparecapture.vi"("error in (no error)"=w749, "Capture mode"=w752, "Handle in"=w748) -> ("error out"=w750:errorcluster, "Handle out"=w751:u32)  [unwired: 5 in, 2 out]
                n86 = call <userlib>:"tm_startcapture_b.vi"("error in (no error)"=w750, "Handle in"=w751) -> ("error out"=w746:errorcluster, "Handle out"=w747:u32)  [unwired: 8 in]
              }
              event "Camera Readout Mode", "Slit Width / Lines": Value Change {
                w769 = 1 items=["Snap", "Sequence"] ("Capture mode")
                n87 = event-data() -> ()  [unwired: 1 in, 4 out]
                n88 = call <userlib>:"tm_stopcapture.vi"("error in (no error)"=w775, "Handle in"=w776) -> ("error out"=w777:errorcluster, "Handle out"=w773:u32)  [unwired: 8 in]
                n89 = call <userlib>:"tm_unpreparecapture.vi"("error in (no error)"=w777, "Handle in"=w773) -> ("error out"=w768:errorcluster, "Handle out"=w774:u32)  [unwired: 8 in]
                n90 = call <userlib>:"tm_setpropertyvalue.vi"("error in (no error)"=w768, "Value in"="Camera Readout Mode", "Property ID"=u32 4194832, "Handle in"=w774) -> ("error out"=w778:errorcluster, "Handle out"=w779:u32)  [unwired: 6 in]
                n91 = case shown="12" "Camera Readout Mode" {
                  tunnel: w779 -> [w790 w797]
                  tunnel: [w789 w792] -> w772
                  tunnel: w778 -> [w787 w802]
                  tunnel: [w786 w802] -> w770
                  frame 1, Default {
                    n92 = local read "Exposure"() -> (w788:dbl)
                    n93 = call <userlib>:"tm_setpropertyvalue.vi"("error in (no error)"=w787, "Value in"=w788, "Property ID"=u32 2031888, "Handle in"=w790) -> ("error out"=w786:errorcluster, "Handle out"=w789:u32)  [unwired: 6 in]
                  }
                  frame 12 {
                    n94 = local read "Exposure"() -> (w801:dbl)
                    n95 = local read "SVW"() -> (w799:i32)
                    n96 = formula code="slitExpos=frameInter*LW/(LinesToReadout\n+10+LW);\nlineInter = slitExpos / LW;"("frameInter"=w801, "LW"="Slit Width / Lines", "LinesToReadout"=w799) -> ("slitExpos"=w793:dbl, "lineInter"=w796:dbl)
                    n97 = call <userlib>:"tm_setpropertyvalue.vi"("Value in"=w796, "Property ID"=u32 4208720, "Handle in"=w797) -> ("Handle out"=w795:u32)  [unwired: 7 in, 1 out]
                    n98 = call <userlib>:"tm_setpropertyvalue.vi"("Value in"=w793, "Property ID"=u32 2031888, "Handle in"=w795) -> ("Handle out"=w792:u32)  [unwired: 7 in, 1 out]
                  }
                }
                n99 = call <userlib>:"tm_preparecapture.vi"("error in (no error)"=w770, "Capture mode"=w769, "Handle in"=w772) -> ("error out"=w765:errorcluster, "Buffer Info"=w771:T7, "Handle out"=w767:u32)  [unwired: 5 in, 1 out]
                n100 = call <userlib>:"tm_startcapture_b.vi"("error in (no error)"=w765, "Handle in"=w767) -> ("error out"=w764:errorcluster, "Handle out"=w766:u32)  [unwired: 8 in]
              }
              event "Ram Record": Value Change {
                n101 = event-data() -> ()  [unwired: 1 in, 5 out]
                n102 = case shown="True" "Ram Record" {
                  tunnel: w816 -> [w820 w843]
                  tunnel: w815 -> [w819 w840]
                  tunnel: [w820 w826] -> w814
                  tunnel: [w819 w828] -> w813
                  tunnel: [w818 w827] -> w809
                  tunnel: w808 -> [w818 _]
                  tunnel: w806 -> [_ w831]
                  tunnel: [_ w829] -> w805
                  tunnel: w804 -> [_ w825]
                  tunnel: w803 -> [_ w821]
                  frame False {
                  }
                  frame True {
                    w837 = 0 items=["Snap", "Sequence"] ("Capture mode")
                    # "Max 2500"
                    n103 = Flush Queue(queue=w831) -> (queue out=w830:refnum<queue>)  [unwired: 1 in, 2 out]
                    n104 = call <userlib>:"tm_stopcapture.vi"("error in (no error)"=w843, "Handle in"=w840) -> ("error out"=w842:errorcluster, "Handle out"=w841:u32)  [unwired: 8 in]
                    n105 = Bundle By Name(cluster=w821, "State"=Stack_Track."Start Sequence", "Stack Number"=0, "Image"=w825) -> (w822:T3)
                    n106 = call <userlib>:"tm_unpreparecapture.vi"("error in (no error)"=w842, "Handle in"=w841) -> ("error out"=w838:errorcluster, "Handle out"=w839:u32)  [unwired: 8 in]
                    n107 = call <userlib>:"tm_preparecapture.vi"("error in (no error)"=w838, "Frames"="Frames", "Capture mode"=w837, "Handle in"=w839) -> ("error out"=w836:errorcluster, "Buffer Info"=w834:T7, "Handle out"=w835:u32)  [unwired: 4 in, 1 out]
                    n108 = Enqueue Element(queue=w830, element=w822) -> (queue out=w832:refnum<queue>)  [unwired: 2 in, 2 out]
                    n109 = case shown="No Error" w836 {
                      selector: w836 -> [w868 w889]
                      tunnel: w835 -> [w867 w890]
                      tunnel: "Frames" -> [w863 _]
                      tunnel: [w848 w886] -> w828
                      tunnel: w834 -> [w864 _]
                      tunnel: [w847 w888] -> w826
                      tunnel: w832 -> [w862 w884]
                      tunnel: w821 -> [w861 _]
                      tunnel: [w846 w884] -> _
                      tunnel: [FALSE ("value") w898] -> w829
                      tunnel: [w845 w887] -> w827
                      frame No Error {
                        w853 = 1 items=["Snap", "Sequence"] ("Capture mode")
                        # "Frames in RAM"
                        n110 = call <userlib>:"tm_startcapture_b.vi"("error in (no error)"=w868, "Handle in"=w867) -> ("error out"=w865:errorcluster, "Handle out"=w866:u32)  [unwired: 8 in]
                        n111 = for {
                          N: w863 -> [_]
                          tunnel: w866 -> [w883]
                          tunnel: w865 -> [w882]
                          tunnel: w864 -> [w879]
                          tunnel: [w878] -> w859
                          tunnel: [w877] -> w858
                          tunnel: w862 -> [w875]
                          tunnel: Stack_Track."Collecting" ("Enum") -> [w873]
                          tunnel: w861 -> [w871]
                          tunnel: [w870] -> w852
                          i -> [w872]
                          n112 = call <userlib>:"tm_waitnextframe.vi"("error in (no error)"=w882, "Handle in"=w883) -> ("error out"=w880:errorcluster, "Frame Index"=→"Frame Index":i32, "Handle out"=w881:u32)  [unwired: 6 in, 1 out]
                          n113 = call <userlib>:"tm_getframe_a.vi"("error in (no error)"=w880, "Frame Index"=w872, "Buffer Info"=w879, "Handle in"=w881) -> ("error out"=w877:errorcluster, "Data 16"=w869:u16[][], "Handle out"=w878:u32)  [unwired: 3 in, 2 out]
                          n114 = Bundle By Name(cluster=w871, "State"=w873, "Stack Number"=w872, "Image"=w869) -> (w874:T3)
                          n115 = Enqueue Element(queue=w875, element=w874) -> (queue out=w870:refnum<queue>)  [unwired: 2 in, 2 out]
                        }
                        n116 = call <userlib>:"tm_stopcapture.vi"("error in (no error)"=w858, "Handle in"=w859) -> ("error out"=w856:errorcluster, "Handle out"=w857:u32)  [unwired: 8 in]
                        n117 = call <userlib>:"tm_unpreparecapture.vi"("error in (no error)"=w856, "Handle in"=w857) -> ("error out"=w855:errorcluster, "Handle out"=w854:u32)  [unwired: 8 in]
                        n118 = Enqueue Element(queue=w852, element=T3 {"State"=enum."End", "Stack Number"=0, "Image"=[]} ("input cluster")) -> (queue out=w846:refnum<queue>)  [unwired: 2 in, 2 out]
                        n119 = call <userlib>:"tm_preparecapture.vi"("error in (no error)"=w855, "Capture mode"=w853, "Handle in"=w854) -> ("error out"=w850:errorcluster, "Buffer Info"=w845:T7, "Handle out"=w849:u32)  [unwired: 5 in, 1 out]
                        n120 = call <userlib>:"tm_startcapture_b.vi"("error in (no error)"=w850, "Handle in"=w849) -> ("error out"=w847:errorcluster, "Handle out"=w848:u32)  [unwired: 8 in]
                      }
                      frame Error {
                        w893 = 1 items=["Snap", "Sequence"] ("Capture mode")
                        # "Prepare camera failure, likely too many frames in stack"
                        n121 = One Button Dialog(message="Too many frames in stack", button name ("OK")="OK") -> (true=w898:bool)
                        n122 = call <userlib>:"tm_stopcapture.vi"("error in (no error)"=w889, "Handle in"=w890) -> ("error out"=w896:errorcluster, "Handle out"=w897:u32)  [unwired: 8 in]
                        n123 = call <userlib>:"tm_unpreparecapture.vi"("error in (no error)"=w896, "Handle in"=w897) -> ("error out"=w895:errorcluster, "Handle out"=w894:u32)  [unwired: 8 in]
                        n124 = Enqueue Element(queue=w884, element=T3 {"State"=enum."Idle", "Stack Number"=0, "Image"=[]} ("input cluster")) -> ()  [unwired: 2 in, 3 out]
                        n125 = call <userlib>:"tm_preparecapture.vi"("error in (no error)"=w895, "Capture mode"=w893, "Handle in"=w894) -> ("error out"=w892:errorcluster, "Buffer Info"=w887:T7, "Handle out"=w891:u32)  [unwired: 5 in, 1 out]
                        n126 = call <userlib>:"tm_startcapture_b.vi"("error in (no error)"=w892, "Handle in"=w891) -> ("error out"=w888:errorcluster, "Handle out"=w886:u32)  [unwired: 8 in]
                      }
                    }
                  }
                }
              }
              event "HardDisk Record": Value Change {
                n127 = event-data() -> ()  [unwired: 1 in, 5 out]
                n128 = case shown="True" "HardDisk Record" {
                  tunnel: w913 -> [w916 w932]
                  tunnel: w912 -> [w915 w929]
                  tunnel: [w916 w919] -> w911
                  tunnel: [w915 w921] -> w910
                  tunnel: [w914 w920] -> w906
                  tunnel: w905 -> [w914 _]
                  tunnel: w903 -> [_ w917]
                  tunnel: [_ w922] -> w902
                  frame False {
                  }
                  frame True {
                    w926 = 0 items=["Snap", "Sequence"] ("Capture mode")
                    # "Max 50"
                    n129 = call <userlib>:"tm_stopcapture.vi"("error in (no error)"=w932, "Handle in"=w929) -> ("error out"=w931:errorcluster, "Handle out"=w930:u32)  [unwired: 8 in]
                    n130 = call <userlib>:"tm_unpreparecapture.vi"("error in (no error)"=w931, "Handle in"=w930) -> ("error out"=w927:errorcluster, "Handle out"=w928:u32)  [unwired: 8 in]
                    n131 = call <userlib>:"tm_preparecapture.vi"("error in (no error)"=w927, "Frames"="Frames", "Capture mode"=w926, "Handle in"=w928) -> ("error out"=w925:errorcluster, "Buffer Info"=w923:T7, "Handle out"=w924:u32)  [unwired: 4 in, 1 out]
                    n132 = case shown="No Error" w925 {
                      selector: w925 -> [w957 w970]
                      tunnel: w924 -> [w943 w971]
                      tunnel: [w946 w967] -> w921
                      tunnel: w923 -> [w954 _]
                      tunnel: [w945 w969] -> w919
                      tunnel: [FALSE ("value") w979] -> w922
                      tunnel: [w944 w968] -> w920
                      tunnel: "Frames" -> [w940 _]
                      tunnel: w917 -> [w934 w965]
                      frame No Error {
                        w949 = 1 items=["Snap", "Sequence"] ("Capture mode")
                        n133 = call <userlib>:"tm_startrecorder.vi"("frames"=w940, "File"="Temp", "Handle in"=w943) -> ("Handle out"=w942:u32)  [unwired: 7 in, 1 out]
                        n134 = call <userlib>:"tm_startcapture_b.vi"("error in (no error)"=w957, "Handle in"=w942) -> ("error out"=w955:errorcluster, "Handle out"=w956:u32)  [unwired: 8 in]
                        n135 = while {
                          tunnel: w956 -> [w963]
                          tunnel: w955 -> [w962]
                          tunnel: w954 -> [_]
                          tunnel: [w964] -> w952
                          tunnel: w940 -> [w959]
                          stop <- w960 stop-if-true
                          n136 = Wait (ms)(milliseconds to wait=u32 50) -> ()  [unwired: 1 out]
                          n137 = call <userlib>:"tm_getrecorderstatus.vi"("error in (no error)"=w962, "Handle"=w963) -> ("error out"=w964:errorcluster, "Count"=w958:i32)  [unwired: 6 in, 2 out]
                          n138 = Equal?(x=w958, y=w959) -> (x = y?=w960:bool)
                        }
                        n139 = call <userlib>:"tm_stopcapture.vi"("error in (no error)"=w952) -> ("error out"=w939:errorcluster, "Handle out"=w938:u32)  [unwired: 9 in]
                        n140 = call <userlib>:"tm_stoprecorder.vi"("error in (no error)"=w939, "Handle in"=w938) -> ("error out"=w936:errorcluster, "Handle out"=w937:u32)  [unwired: 8 in]
                        n141 = Enqueue Element(queue=w934, element=T3 {"State"=enum."Read Disk", "Stack Number"=0, "Image"=[]}, error in (no error)=w936) -> (error out=w935:errorcluster)  [unwired: 1 in, 2 out]
                        n142 = call <userlib>:"tm_unpreparecapture.vi"("error in (no error)"=w935, "Handle in"=w937) -> ("error out"=w951:errorcluster, "Handle out"=w950:u32)  [unwired: 8 in]
                        n143 = call <userlib>:"tm_preparecapture.vi"("error in (no error)"=w951, "Capture mode"=w949, "Handle in"=w950) -> ("error out"=w948:errorcluster, "Buffer Info"=w944:T7, "Handle out"=w947:u32)  [unwired: 5 in, 1 out]
                        n144 = call <userlib>:"tm_startcapture_b.vi"("error in (no error)"=w948, "Handle in"=w947) -> ("error out"=w945:errorcluster, "Handle out"=w946:u32)  [unwired: 8 in]
                      }
                      frame Error {
                        w974 = 1 items=["Snap", "Sequence"] ("Capture mode")
                        # "Prepare camera failure, likely too many frames in stack"
                        n145 = One Button Dialog(message="Too many frames in stack", button name ("OK")="OK") -> (true=w979:bool)
                        n146 = call <userlib>:"tm_stopcapture.vi"("error in (no error)"=w970, "Handle in"=w971) -> ("error out"=w977:errorcluster, "Handle out"=w978:u32)  [unwired: 8 in]
                        n147 = call <userlib>:"tm_unpreparecapture.vi"("error in (no error)"=w977, "Handle in"=w978) -> ("error out"=w976:errorcluster, "Handle out"=w975:u32)  [unwired: 8 in]
                        n148 = Enqueue Element(queue=w965, element=T3 {"State"=enum."STOP", "Stack Number"=0, "Image"=[]} ("input cluster")) -> ()  [unwired: 2 in, 3 out]
                        n149 = call <userlib>:"tm_preparecapture.vi"("error in (no error)"=w976, "Capture mode"=w974, "Handle in"=w975) -> ("error out"=w973:errorcluster, "Buffer Info"=w968:T7, "Handle out"=w972:u32)  [unwired: 5 in, 1 out]
                        n150 = call <userlib>:"tm_startcapture_b.vi"("error in (no error)"=w973, "Handle in"=w972) -> ("error out"=w969:errorcluster, "Handle out"=w967:u32)  [unwired: 8 in]
                      }
                    }
                  }
                }
              }
              event "Scan Mode": Value Change {
                w982 = u32 4211872 items=["SENSOR MODE"=4212128, "CCD MODE"=4212384, "READOUT MODE"=4211872, "ACTIVE VIEW INDEX"=4343136, "BITS PER CHANNEL"=4342976, "IMAGE PIXEL TYPE"=4343296, "BINNING"=4215968, "EXPOSURE TIME"=2049184, "CONTRAST GAIN"=3163312, "CONTRAST OFFSET"=3163328, "LIGHT MODE"=2114720, "SENSITIVITY"=2114992, "PHOTON IMAGING MODE"=2115200, "HIGH DYNAMIC RANGE MODE"=3163360, "WHITE BALANCE"=3163568, "TEMPERATURE"=2115232, "TEMPERATURE TARGET"=2115264, "SENSOR COOLER FAN"=2115296, "LINEBUNDLE HEIGHT"=4212192, "MECHANICAL SHUTTER"=2115488, "BACK FOCUS POSITION"=8422304, "TRIGGER CONNECTOR"=1066432, "TRIGGER SOURCE"=1066144, "OUTPUT TRIGGER SOURCE"=1852576, "TRIGGER GLOBAL EXPOSURE"=2049680, "FIRST TRIGGER BEHAVIOR"=2049696, "CHANNEL SYNC"=1852352, "READOUT DIRECTION"=4211904, "PRE HSYNC COUNT"=1852704] ("Parameter")
                w997 = 1 items=["Snap", "Sequence"] ("Capture mode")
                n151 = event-data() -> ("NewVal"=w987:dbl)  [unwired: 1 in, 2 out]
                n152 = call <userlib>:"tm_stopcapture.vi"("error in (no error)"=w998, "Handle in"=w999) -> ("error out"=w1000:errorcluster, "Handle out"=w1001:u32)  [unwired: 8 in]
                n153 = call <userlib>:"tm_unpreparecapture.vi"("error in (no error)"=w1000, "Handle in"=w1001) -> ("error out"=w985:errorcluster, "Handle out"=w986:u32)  [unwired: 8 in]
                n154 = call <userlib>:"tm_setparameter_a.vi"("error in (no error)"=w985, "Value in"=w987, "Parameter"=w982, "Handle in"=w986) -> ("error out"=w984:errorcluster, "Handle out"=w983:u32)  [unwired: 6 in]
                n155 = call <userlib>:"tm_getparameter_a.vi"("error in (no error)"=w984, "Parameter"=w982, "Handle in"=w983) -> ("error out"=w990:errorcluster, "Value out"=w989:dbl, "Handle out"=w988:u32)  [unwired: 6 in]
                n156 = local write "SMD"(w989) -> ()
                n157 = call <userlib>:"tm_preparecapture.vi"("error in (no error)"=w990, "Capture mode"=w997, "Handle in"=w988) -> ("error out"=w995:errorcluster, "Buffer Info"=w992:T7, "Handle out"=w996:u32)  [unwired: 5 in, 1 out]
                n158 = call <userlib>:"tm_startcapture_b.vi"("error in (no error)"=w995, "Handle in"=w996) -> ("error out"=w994:errorcluster, "Handle out"=w993:u32)  [unwired: 8 in]
              }
              event "Binning": Value Change {
                w1006 = u32 4215968 items=["BINNING"=4215968, "BITS PER CHANNEL"=2, "ACTIVE VIEW INDEX"=3, "CCD MODE"=4, "SENSOR MODE"=5, "READOUT MODE"=6, "EXPOSURE TIME"=7, "CONTRAST GAIN"=8, "CONTRAST OFFSET"=9, "LIGHT MODE"=10, "SENSITIVITY"=11, "WHITE BALANCE"=12, "PHOTON IMAGING MODE"=13, "HIGH DYNAMIC RANGE MODE"=14, "TRIGGER SOURCE"=15, "TRIGGER ACTIVE"=16, "TRIGGER MODE"=17, "TRIGGER POLARITY"=18, "TRIGGER GLOBAL EXPOSURE"=19, "FIRST TRIGGER BEHAVIOR"=20, "TRIGGER TIMES"=21, "OUTPUT TRIGGER POLARITY"=22, "OUTPUT TRIGGER DELAY"=23, "OUTPUT TRIGGER PERIOD"=24, "TEMPERATURE"=25, "TEMPERATURE TARGET"=26, "SENSOR COOLER FAN"=27, "MECHANICAL SHUTTER"=28, "BACK FOCUS POSITION"=29, "FRAMEBUNDLE MODE"=30, "FRAMEBUNDLE NUMBER"=31, "LINEBUNDLE HEIGHT"=32, "TRIGGER CONNECTOR"=33, "IMAGE PIXEL TYPE"=34, "OUTPUT TRIGGER KIND"=35, "READOUT DIRECTION"=36, "CHANNEL SYNC"=37] ("Parameter")
                w1045 = 1 items=["Snap", "Sequence"] ("Capture mode")
                n159 = event-data() -> ("NewVal"=w1007:u16)  [unwired: 1 in, 2 out]
                n160 = call <userlib>:"tm_stopcapture.vi"("error in (no error)"=w1014, "Handle in"=w1015) -> ("error out"=w1012:errorcluster, "Handle out"=w1013:u32)  [unwired: 8 in]
                n161 = call <userlib>:"tm_unpreparecapture.vi"("error in (no error)"=w1012, "Handle in"=w1013) -> ("error out"=w1008:errorcluster, "Handle out"=w1005:u32)  [unwired: 8 in]
                n162 = call <userlib>:"tm_setparameter_a.vi"("error in (no error)"=w1008, "Value in"=w1007, "Parameter"=w1006, "Handle in"=w1005) -> ("error out"=w1009:errorcluster, "Handle out"=w1010:u32)  [unwired: 6 in]
                n163 = call <userlib>:"tm_getarea_a.vi"("error in (no error)"=w1009, "Handle in"=w1010) -> ("error out"=w1033:errorcluster, "V Offset"=w1035:T6, "H Offset"=w1034:T6, "Handle out"=w1032:u32, "H Width"=w1036:T6, "V Width"=w1037:T6)  [unwired: 4 in]
                n164 = Unbundle By Name(w1034) -> ("Value"=w1028:i32, "Minimum"=w1031:i32, "Maximum"=w1030:i32, "Increment"=w1029:i32)
                n165 = Unbundle By Name(w1035) -> ("Value"=w1018:i32, "Minimum"=w1027:i32, "Maximum"=w1026:i32, "Increment"=w1025:i32)
                n166 = Unbundle By Name(w1036) -> ("Value"=w1017:i32, "Minimum"=w1024:i32, "Maximum"=w1023:i32, "Increment"=w1022:i32)
                n167 = Unbundle By Name(w1037) -> ("Value"=w1016:i32, "Minimum"=w1021:i32, "Maximum"=w1020:i32, "Increment"=w1019:i32)
                n168 = property on="H Offset" class="DigNum (strict)"("Value"=w1028, "Minimum"=w1031, "Maximum"=w1030, "Increment"=w1029) -> ()  [unwired: 2 in, 2 out]
                n169 = property on="V Offset" class="DigNum (strict)"("Value"=w1018, "Minimum"=w1027, "Maximum"=w1026, "Increment"=w1025) -> ()  [unwired: 2 in, 2 out]
                n170 = property on="H Width" class="DigNum (strict)"("Value"=w1017, "Minimum"=w1024, "Maximum"=w1023, "Increment"=w1022) -> ()  [unwired: 2 in, 2 out]
                n171 = property on="V Width" class="DigNum (strict)"("Value"=w1016, "Minimum"=w1021, "Maximum"=w1020, "Increment"=w1019) -> ()  [unwired: 2 in, 2 out]
                n172 = local write "SHO"(w1028) -> ()
                n173 = local write "SVO"(w1018) -> ()
                n174 = local write "SHW"(w1017) -> ()
                n175 = local write "SVW"(w1016) -> ()
                n176 = call <userlib>:"tm_preparecapture.vi"("error in (no error)"=w1033, "Capture mode"=w1045, "Handle in"=w1032) -> ("error out"=w1043:errorcluster, "Buffer Info"=w1040:T7, "Handle out"=w1044:u32)  [unwired: 5 in, 1 out]
                n177 = call <userlib>:"tm_startcapture_b.vi"("error in (no error)"=w1043, "Handle in"=w1044) -> ("error out"=w1042:errorcluster, "Handle out"=w1041:u32)  [unwired: 8 in]
              }
              event "H Offset", "H Width", "V Offset", "V Width": Value Change {
                w1090 = 1 items=["Snap", "Sequence"] ("Capture mode")
                n178 = event-data() -> ()  [unwired: 1 in, 4 out]
                n179 = call <userlib>:"tm_stopcapture.vi"("error in (no error)"=w1052, "Handle in"=w1053) -> ("error out"=w1050:errorcluster, "Handle out"=w1051:u32)  [unwired: 8 in]
                n180 = local read "H Offset"() -> (w1056:i32)
                n181 = local read "H Width"() -> (w1057:i32)
                n182 = local read "V Offset"() -> (w1058:i32)
                n183 = local read "V Width"() -> (w1055:i32)
                n184 = call <userlib>:"tm_unpreparecapture.vi"("error in (no error)"=w1050, "Handle in"=w1051) -> ("error out"=w1048:errorcluster, "Handle out"=w1049:u32)  [unwired: 8 in]
                n185 = Bundle("H Offset"=w1056, "V Offset"=w1058, "H Width"=w1057, "V Width"=w1055) -> (w1054:T8)  [unwired: 1 in]
                n186 = call <userlib>:"tm_setarea.vi"("error in (no error)"=w1048, "Sub Region"=w1054, "Handle in"=w1049) -> ("error out"=w1059:errorcluster, "Handle out"=w1060:u32)  [unwired: 7 in]
                n187 = call <userlib>:"tm_getarea_a.vi"("error in (no error)"=w1059, "Handle in"=w1060) -> ("error out"=w1078:errorcluster, "V Offset"=w1080:T6, "H Offset"=w1079:T6, "Handle out"=w1077:u32, "H Width"=w1081:T6, "V Width"=w1082:T6)  [unwired: 4 in]
                n188 = Unbundle By Name(w1079) -> ("Value"=w1073:i32, "Minimum"=w1076:i32, "Maximum"=w1075:i32, "Increment"=w1074:i32)
                n189 = Unbundle By Name(w1080) -> ("Value"=w1063:i32, "Minimum"=w1072:i32, "Maximum"=w1071:i32, "Increment"=w1070:i32)
                n190 = Unbundle By Name(w1081) -> ("Value"=w1062:i32, "Minimum"=w1069:i32, "Maximum"=w1068:i32, "Increment"=w1067:i32)
                n191 = Unbundle By Name(w1082) -> ("Value"=w1061:i32, "Minimum"=w1066:i32, "Maximum"=w1065:i32, "Increment"=w1064:i32)
                n192 = property on="H Offset" class="DigNum (strict)"("Value"=w1073, "Minimum"=w1076, "Maximum"=w1075, "Increment"=w1074) -> ()  [unwired: 2 in, 2 out]
                n193 = property on="V Offset" class="DigNum (strict)"("Value"=w1063, "Minimum"=w1072, "Maximum"=w1071, "Increment"=w1070) -> ()  [unwired: 2 in, 2 out]
                n194 = property on="H Width" class="DigNum (strict)"("Value"=w1062, "Minimum"=w1069, "Maximum"=w1068, "Increment"=w1067) -> ()  [unwired: 2 in, 2 out]
                n195 = property on="V Width" class="DigNum (strict)"("Value"=w1061, "Minimum"=w1066, "Maximum"=w1065, "Increment"=w1064) -> ()  [unwired: 2 in, 2 out]
                n196 = local write "SHO"(w1073) -> ()
                n197 = local write "SVO"(w1063) -> ()
                n198 = local write "SHW"(w1062) -> ()
                n199 = local write "SVW"(w1061) -> ()
                n200 = call <userlib>:"tm_preparecapture.vi"("error in (no error)"=w1078, "Capture mode"=w1090, "Handle in"=w1077) -> ("error out"=w1088:errorcluster, "Buffer Info"=w1085:T7, "Handle out"=w1089:u32)  [unwired: 5 in, 1 out]
                n201 = call <userlib>:"tm_startcapture_b.vi"("error in (no error)"=w1088, "Handle in"=w1089) -> ("error out"=w1087:errorcluster, "Handle out"=w1086:u32)  [unwired: 8 in]
              }
            }
            n202 = local read "stop"() -> (w594:bool)
            n203 = Unbundle By Name(w603) -> ("status"=w616:bool)
            n204 = Compound Arithmetic op=OR(w616, w594, w598) -> (w615:bool)
          }
        }
        frame Enabled {
        }
      }
      n205 = while {
        tunnel: w14 -> [w172]
        tunnel: w17 -> [w175]
        tunnel: w28 -> [w171]
        shift-right: [w170] -> _
        shift-left: w27 -> [w173]
        shift-right: [w169] -> w23
        shift-left: w26 -> [w174]
        tunnel: w25 -> [w168]
        tunnel: [w162] -> w22
        shift-right: [w160] -> _
        shift-left: _ -> [w159]
        shift-right: [w158] -> _
        shift-left: CameraControlTypeDef."Preview" ("Enum") -> [w157]
        stop <- w161 stop-if-true
        n206 = Dequeue Element(queue=w175, timeout in ms (-1)=1) -> (element=w164:T2, timed out?=w166:bool)  [unwired: 1 in, 2 out]
        n207 = case shown="True" w166 {
          tunnel: [w176 w177] -> w165
          tunnel: w164 -> [w176 _]
          tunnel: w157 -> [_ w177]
          frame False {
          }
          frame True {
          }
        }
        n208 = case shown="\"Ram Record\"" w165 {
          tunnel: w174 -> [w199 w281 w334 w377 w417 w455 w490 w494 w512 w522 w556 w577 w581]
          tunnel: w173 -> [_ _ _ _ _ w462 w484 w495 _ _ _ _ w580]
          tunnel: w172 -> [w201 w282 _ _ _ _ w489 _ _ _ _ _ _]
          tunnel: w171 -> [w202 _ _ _ _ _ w488 _ _ _ _ _ _]
          tunnel: [w198 w277 w347 w386 w424 w462 w484 w495 w498 w520 w540 w561 w580] -> w170
          tunnel: [w197 w278 w340 w384 w422 w463 w483 w494 w502 w519 w552 w573 w581] -> w169
          tunnel: w168 -> [w200 w280 w372 w412 w432 w454 w481 w493 w515 w521 w546 w567 w582]
          tunnel: [w196 w279 w346 w385 w423 w461 w482 w493 w503 w518 w551 w572 w582] -> w162
          tunnel: [w180 w266 w333 w376 w416 w453 w480 w492 w497 w517 w538 w559 w579] -> w160
          tunnel: w159 -> [w179 w266 w333 w376 w416 w453 _ w492 w497 w517 w538 w559 w579]
          tunnel: [w178 w265 w332 w375 w415 w452 CameraControlTypeDef."Preview" ("Enum") CameraControlTypeDef."Idle" ("Enum") w496 w516 w537 w558 w578] -> w158
          tunnel: w157 -> [w178 w265 w332 w375 w415 w452 _ _ w496 w516 w537 w558 w578]
          frame "Ram Record" {
            w191 = 0 items=["Snap", "Sequence"] ("Capture mode")
            # "Max 2500"
            n209 = local read "Stack Frames"() -> (w182:i32)
            n210 = Flush Queue(queue=w201) -> (queue out=w186:refnum<queue>)  [unwired: 1 in, 2 out]
            n211 = call <userlib>:"tm_stopcapture.vi"("error in (no error)"=w200, "Handle in"=w199) -> ("error out"=w195:errorcluster, "Handle out"=w194:u32)  [unwired: 8 in]
            n212 = Bundle By Name(cluster=w202, "State"=Stack_Track."Start Sequence", "Stack Number"=0, "Image"=w179) -> (w183:T3)
            n213 = call <userlib>:"tm_unpreparecapture.vi"("error in (no error)"=w195, "Handle in"=w194) -> ("error out"=w192:errorcluster, "Handle out"=w193:u32)  [unwired: 8 in]
            n214 = call <userlib>:"tm_preparecapture.vi"("error in (no error)"=w192, "Frames"=w182, "Capture mode"=w191, "Handle in"=w193) -> ("error out"=w190:errorcluster, "Buffer Info"=w188:T7, "Handle out"=w189:u32)  [unwired: 4 in, 1 out]
            n215 = Enqueue Element(queue=w186, element=w183) -> (queue out=w187:refnum<queue>)  [unwired: 2 in, 2 out]
            n216 = case shown="No Error" w190 {
              selector: w190 -> [w230 w253]
              tunnel: w189 -> [w229 w254]
              tunnel: w182 -> [w225 _]
              tunnel: [w210 w250] -> w197
              tunnel: w188 -> [w226 _]
              tunnel: [w209 w252] -> w196
              tunnel: w187 -> [w224 w248]
              tunnel: w202 -> [w223 _]
              tunnel: [w208 w248] -> _
              tunnel: [FALSE ("value") w262] -> _
              tunnel: [w207 w251] -> w198
              tunnel: [FALSE ("Boolean") _] -> w181
              tunnel: [w204 w247] -> w180
              tunnel: w179 -> [_ w247]
              frame No Error {
                w215 = 1 items=["Snap", "Sequence"] ("Capture mode")
                # "Frames in RAM"
                n217 = call <userlib>:"tm_startcapture_b.vi"("error in (no error)"=w230, "Handle in"=w229) -> ("error out"=w227:errorcluster, "Handle out"=w228:u32)  [unwired: 8 in]
                n218 = for {
                  N: w225 -> [_]
                  tunnel: w228 -> [w246]
                  tunnel: w227 -> [w245]
                  tunnel: w226 -> [w242]
                  tunnel: [w241] -> w221
                  tunnel: [w240] -> w220
                  tunnel: w224 -> [w239]
                  tunnel: Stack_Track."Collecting" ("Enum") -> [w237]
                  tunnel: w223 -> [w235]
                  tunnel: [w234] -> w214
                  tunnel: [w232] -> w204
                  tunnel: TRUE ("Boolean") -> [w231]
                  i -> [w236]
                  n219 = local write "Record Ready"(w231) -> ()
                  n220 = call <userlib>:"tm_waitnextframe.vi"("error in (no error)"=w245, "Handle in"=w246) -> ("error out"=w243:errorcluster, "Frame Index"=w233:i32, "Handle out"=w244:u32)  [unwired: 6 in, 1 out]
                  n221 = call <userlib>:"tm_getframe_a.vi"("error in (no error)"=w243, "Frame Index"=w236, "Buffer Info"=w242, "Handle in"=w244) -> ("error out"=w240:errorcluster, "Data 16"=w232:u16[][], "Handle out"=w241:u32)  [unwired: 3 in, 2 out]
                  n222 = Bundle By Name(cluster=w235, "State"=w237, "Stack Number"=w236, "Image"=w232) -> (w238:T3)
                  n223 = Enqueue Element(queue=w239, element=w238) -> (queue out=w234:refnum<queue>)  [unwired: 2 in, 2 out]
                  n224 = local write "Stack Frames"(w233) -> ()
                }
                n225 = call <userlib>:"tm_stopcapture.vi"("error in (no error)"=w220, "Handle in"=w221) -> ("error out"=w218:errorcluster, "Handle out"=w219:u32)  [unwired: 8 in]
                n226 = call <userlib>:"tm_unpreparecapture.vi"("error in (no error)"=w218, "Handle in"=w219) -> ("error out"=w217:errorcluster, "Handle out"=w216:u32)  [unwired: 8 in]
                n227 = Enqueue Element(queue=w214, element=T3 {"State"=enum."End", "Stack Number"=0, "Image"=[]} ("input cluster")) -> (queue out=w208:refnum<queue>)  [unwired: 2 in, 2 out]
                n228 = call <userlib>:"tm_preparecapture.vi"("error in (no error)"=w217, "Capture mode"=w215, "Handle in"=w216) -> ("error out"=w212:errorcluster, "Buffer Info"=w207:T7, "Handle out"=w211:u32)  [unwired: 5 in, 1 out]
                n229 = call <userlib>:"tm_startcapture_b.vi"("error in (no error)"=w212, "Handle in"=w211) -> ("error out"=w209:errorcluster, "Handle out"=w210:u32)  [unwired: 8 in]
              }
              frame Error {
                w257 = 1 items=["Snap", "Sequence"] ("Capture mode")
                # "Prepare camera failure, likely too many frames in stack"
                n230 = One Button Dialog(message="Too many frames in stack", button name ("OK")="OK") -> (true=w262:bool)
                n231 = call <userlib>:"tm_stopcapture.vi"("error in (no error)"=w253, "Handle in"=w254) -> ("error out"=w260:errorcluster, "Handle out"=w261:u32)  [unwired: 8 in]
                n232 = call <userlib>:"tm_unpreparecapture.vi"("error in (no error)"=w260, "Handle in"=w261) -> ("error out"=w259:errorcluster, "Handle out"=w258:u32)  [unwired: 8 in]
                n233 = Enqueue Element(queue=w248, element=T3 {"State"=enum."Idle", "Stack Number"=0, "Image"=[]} ("input cluster")) -> ()  [unwired: 2 in, 3 out]
                n234 = call <userlib>:"tm_preparecapture.vi"("error in (no error)"=w259, "Capture mode"=w257, "Handle in"=w258) -> ("error out"=w256:errorcluster, "Buffer Info"=w251:T7, "Handle out"=w255:u32)  [unwired: 5 in, 1 out]
                n235 = call <userlib>:"tm_startcapture_b.vi"("error in (no error)"=w256, "Handle in"=w255) -> ("error out"=w252:errorcluster, "Handle out"=w250:u32)  [unwired: 8 in]
              }
            }
            n236 = local write "Record Ready"(w181) -> ()
          }
          frame "HardDisk Record" {
            w272 = 0 items=["Snap", "Sequence"] ("Capture mode")
            # "Would add for loop here"
            # "Max 50"
            n237 = local read "Stack Frames"() -> (w268:i32)
            n238 = call <userlib>:"tm_stopcapture.vi"("error in (no error)"=w280, "Handle in"=w281) -> ("error out"=w276:errorcluster, "Handle out"=w275:u32)  [unwired: 8 in]
            n239 = call <userlib>:"tm_unpreparecapture.vi"("error in (no error)"=w276, "Handle in"=w275) -> ("error out"=w273:errorcluster, "Handle out"=w274:u32)  [unwired: 8 in]
            n240 = call <userlib>:"tm_preparecapture.vi"("error in (no error)"=w273, "Frames"=w268, "Capture mode"=w272, "Handle in"=w274) -> ("error out"=w271:errorcluster, "Buffer Info"=w269:T7, "Handle out"=w270:u32)  [unwired: 4 in, 1 out]
            n241 = case shown="No Error" w271 {
              selector: w271 -> [w307 w320]
              tunnel: w270 -> [w293 w321]
              tunnel: [w296 w317] -> w278
              tunnel: w269 -> [w304 _]
              tunnel: [w295 w319] -> w279
              tunnel: [FALSE ("value") w329] -> _
              tunnel: [w294 w318] -> w277
              tunnel: w268 -> [w291 _]
              tunnel: w282 -> [w285 w315]
              tunnel: path "C:/temp.tmp" ("Temp 2") -> [w283 _]
              frame No Error {
                w299 = 1 items=["Snap", "Sequence"] ("Capture mode")
                n242 = call <userlib>:"tm_startrecorder.vi"("frames"=w291, "File"=w283, "Handle in"=w293) -> ("Handle out"=w292:u32)  [unwired: 7 in, 1 out]
                n243 = call <userlib>:"tm_startcapture_b.vi"("error in (no error)"=w307, "Handle in"=w292) -> ("error out"=w305:errorcluster, "Handle out"=w306:u32)  [unwired: 8 in]
                n244 = while {
                  tunnel: w306 -> [w313]
                  tunnel: w305 -> [w312]
                  tunnel: w304 -> [_]
                  tunnel: [w314] -> w302
                  tunnel: w291 -> [w309]
                  stop <- w310 stop-if-true
                  n245 = Wait (ms)(milliseconds to wait=u32 50) -> ()  [unwired: 1 out]
                  n246 = call <userlib>:"tm_getrecorderstatus.vi"("error in (no error)"=w312, "Handle"=w313) -> ("error out"=w314:errorcluster, "Count"=w308:i32)  [unwired: 6 in, 2 out]
                  n247 = Equal?(x=w308, y=w309) -> (x = y?=w310:bool)
                }
                n248 = call <userlib>:"tm_stopcapture.vi"("error in (no error)"=w302) -> ("error out"=w290:errorcluster, "Handle out"=w289:u32)  [unwired: 9 in]
                n249 = call <userlib>:"tm_stoprecorder.vi"("error in (no error)"=w290, "Handle in"=w289) -> ("error out"=w287:errorcluster, "Handle out"=w288:u32)  [unwired: 8 in]
                n250 = Enqueue Element(queue=w285, element=T3 {"State"=enum."Read Disk", "Stack Number"=0, "Image"=[]}, error in (no error)=w287) -> (error out=w286:errorcluster)  [unwired: 1 in, 2 out]
                n251 = call <userlib>:"tm_unpreparecapture.vi"("error in (no error)"=w286, "Handle in"=w288) -> ("error out"=w301:errorcluster, "Handle out"=w300:u32)  [unwired: 8 in]
                n252 = call <userlib>:"tm_preparecapture.vi"("error in (no error)"=w301, "Capture mode"=w299, "Handle in"=w300) -> ("error out"=w298:errorcluster, "Buffer Info"=w294:T7, "Handle out"=w297:u32)  [unwired: 5 in, 1 out]
                n253 = call <userlib>:"tm_startcapture_b.vi"("error in (no error)"=w298, "Handle in"=w297) -> ("error out"=w295:errorcluster, "Handle out"=w296:u32)  [unwired: 8 in]
              }
              frame Error {
                w324 = 1 items=["Snap", "Sequence"] ("Capture mode")
                # "Prepare camera failure, likely too many frames in stack"
                n254 = One Button Dialog(message="Too many frames in stack", button name ("OK")="OK") -> (true=w329:bool)
                n255 = call <userlib>:"tm_stopcapture.vi"("error in (no error)"=w320, "Handle in"=w321) -> ("error out"=w327:errorcluster, "Handle out"=w328:u32)  [unwired: 8 in]
                n256 = call <userlib>:"tm_unpreparecapture.vi"("error in (no error)"=w327, "Handle in"=w328) -> ("error out"=w326:errorcluster, "Handle out"=w325:u32)  [unwired: 8 in]
                n257 = Enqueue Element(queue=w315, element=T3 {"State"=enum."STOP", "Stack Number"=0, "Image"=[]} ("input cluster")) -> ()  [unwired: 2 in, 3 out]
                n258 = call <userlib>:"tm_preparecapture.vi"("error in (no error)"=w326, "Capture mode"=w324, "Handle in"=w325) -> ("error out"=w323:errorcluster, "Buffer Info"=w318:T7, "Handle out"=w322:u32)  [unwired: 5 in, 1 out]
                n259 = call <userlib>:"tm_startcapture_b.vi"("error in (no error)"=w323, "Handle in"=w322) -> ("error out"=w319:errorcluster, "Handle out"=w317:u32)  [unwired: 8 in]
              }
            }
          }
          frame "ROI" {
            w350 = 1 items=["Snap", "Sequence"] ("Capture mode")
            n260 = call <userlib>:"tm_stopcapture.vi"("error in (no error)"=w372, "Handle in"=w334) -> ("error out"=w373:errorcluster, "Handle out"=w374:u32)  [unwired: 8 in]
            n261 = call <userlib>:"tm_unpreparecapture.vi"("error in (no error)"=w373, "Handle in"=w374) -> ("error out"=w336:errorcluster, "Handle out"=w337:u32)  [unwired: 8 in]
            n262 = local read "V Width"() -> (w342:i32)
            n263 = local read "V Offset"() -> (w344:i32)
            n264 = local read "H Width"() -> (w343:i32)
            n265 = local read "H Offset"() -> (w345:i32)
            n266 = Bundle("H Offset"=w345, "V Offset"=w344, "H Width"=w343, "V Width"=w342) -> (w341:T8)  [unwired: 1 in]
            n267 = call <userlib>:"tm_setarea.vi"("error in (no error)"=w336, "Sub Region"=w341, "Handle in"=w337) -> ("error out"=w339:errorcluster, "Handle out"=w338:u32)  [unwired: 7 in]
            n268 = call <userlib>:"tm_getarea_a.vi"("error in (no error)"=w339, "Handle in"=w338) -> ("error out"=w351:errorcluster, "V Offset"=w354:T6, "H Offset"=w355:T6, "Handle out"=w335:u32, "H Width"=w353:T6, "V Width"=w352:T6)  [unwired: 4 in]
            n269 = Unbundle By Name(w355) -> ("Value"=w359:i32, "Minimum"=w356:i32, "Maximum"=w357:i32, "Increment"=w358:i32)
            n270 = Unbundle By Name(w354) -> ("Value"=w369:i32, "Minimum"=w360:i32, "Maximum"=w361:i32, "Increment"=w362:i32)
            n271 = Unbundle By Name(w353) -> ("Value"=w370:i32, "Minimum"=w363:i32, "Maximum"=w364:i32, "Increment"=w365:i32)
            n272 = Unbundle By Name(w352) -> ("Value"=w371:i32, "Minimum"=w366:i32, "Maximum"=w367:i32, "Increment"=w368:i32)
            n273 = property on="H Offset" class="DigNum (strict)"("Value"=w359, "Minimum"=w356, "Maximum"=w357, "Increment"=w358) -> ()  [unwired: 2 in, 2 out]
            n274 = property on="V Offset" class="DigNum (strict)"("Value"=w369, "Minimum"=w360, "Maximum"=w361, "Increment"=w362) -> ()  [unwired: 2 in, 2 out]
            n275 = property on="H Width" class="DigNum (strict)"("Value"=w370, "Minimum"=w363, "Maximum"=w364, "Increment"=w365) -> ()  [unwired: 2 in, 2 out]
            n276 = property on="V Width" class="DigNum (strict)"("Value"=w371, "Minimum"=w366, "Maximum"=w367, "Increment"=w368) -> ()  [unwired: 2 in, 2 out]
            n277 = local write "SHO"(w359) -> ()
            n278 = local write "SVO"(w369) -> ()
            n279 = local write "SHW"(w370) -> ()
            n280 = local write "SVW"(w371) -> ()
            n281 = call <userlib>:"tm_preparecapture.vi"("error in (no error)"=w351, "Capture mode"=w350, "Handle in"=w335) -> ("error out"=w349:errorcluster, "Buffer Info"=w347:T7, "Handle out"=w348:u32)  [unwired: 5 in, 1 out]
            n282 = call <userlib>:"tm_startcapture_b.vi"("error in (no error)"=w349, "Handle in"=w348) -> ("error out"=w346:errorcluster, "Handle out"=w340:u32)  [unwired: 8 in]
          }
          frame "Binning" {
            w389 = 1 items=["Snap", "Sequence"] ("Capture mode")
            w379 = u32 4215968 items=["BINNING"=4215968, "BITS PER CHANNEL"=2, "ACTIVE VIEW INDEX"=3, "CCD MODE"=4, "SENSOR MODE"=5, "READOUT MODE"=6, "EXPOSURE TIME"=7, "CONTRAST GAIN"=8, "CONTRAST OFFSET"=9, "LIGHT MODE"=10, "SENSITIVITY"=11, "WHITE BALANCE"=12, "PHOTON IMAGING MODE"=13, "HIGH DYNAMIC RANGE MODE"=14, "TRIGGER SOURCE"=15, "TRIGGER ACTIVE"=16, "TRIGGER MODE"=17, "TRIGGER POLARITY"=18, "TRIGGER GLOBAL EXPOSURE"=19, "FIRST TRIGGER BEHAVIOR"=20, "TRIGGER TIMES"=21, "OUTPUT TRIGGER POLARITY"=22, "OUTPUT TRIGGER DELAY"=23, "OUTPUT TRIGGER PERIOD"=24, "TEMPERATURE"=25, "TEMPERATURE TARGET"=26, "SENSOR COOLER FAN"=27, "MECHANICAL SHUTTER"=28, "BACK FOCUS POSITION"=29, "FRAMEBUNDLE MODE"=30, "FRAMEBUNDLE NUMBER"=31, "LINEBUNDLE HEIGHT"=32, "TRIGGER CONNECTOR"=33, "IMAGE PIXEL TYPE"=34, "OUTPUT TRIGGER KIND"=35, "READOUT DIRECTION"=36, "CHANNEL SYNC"=37] ("Parameter")
            n283 = local read "Binning"() -> (w411:u16)
            n284 = call <userlib>:"tm_stopcapture.vi"("error in (no error)"=w412, "Handle in"=w377) -> ("error out"=w413:errorcluster, "Handle out"=w414:u32)  [unwired: 8 in]
            n285 = call <userlib>:"tm_unpreparecapture.vi"("error in (no error)"=w413, "Handle in"=w414) -> ("error out"=w382:errorcluster, "Handle out"=w383:u32)  [unwired: 8 in]
            n286 = call <userlib>:"tm_setparameter_a.vi"("error in (no error)"=w382, "Value in"=w411, "Parameter"=w379, "Handle in"=w383) -> ("error out"=w380:errorcluster, "Handle out"=w378:u32)  [unwired: 6 in]
            n287 = call <userlib>:"tm_getarea_a.vi"("error in (no error)"=w380, "Handle in"=w378) -> ("error out"=w390:errorcluster, "V Offset"=w393:T6, "H Offset"=w394:T6, "Handle out"=w381:u32, "H Width"=w392:T6, "V Width"=w391:T6)  [unwired: 4 in]
            n288 = Unbundle By Name(w394) -> ("Value"=w398:i32, "Minimum"=w395:i32, "Maximum"=w396:i32, "Increment"=w397:i32)
            n289 = Unbundle By Name(w393) -> ("Value"=w408:i32, "Minimum"=w399:i32, "Maximum"=w400:i32, "Increment"=w401:i32)
            n290 = Unbundle By Name(w392) -> ("Value"=w409:i32, "Minimum"=w402:i32, "Maximum"=w403:i32, "Increment"=w404:i32)
            n291 = Unbundle By Name(w391) -> ("Value"=w410:i32, "Minimum"=w405:i32, "Maximum"=w406:i32, "Increment"=w407:i32)
            n292 = property on="H Offset" class="DigNum (strict)"("Value"=w398, "Minimum"=w395, "Maximum"=w396, "Increment"=w397) -> ()  [unwired: 2 in, 2 out]
            n293 = property on="V Offset" class="DigNum (strict)"("Value"=w408, "Minimum"=w399, "Maximum"=w400, "Increment"=w401) -> ()  [unwired: 2 in, 2 out]
            n294 = property on="H Width" class="DigNum (strict)"("Value"=w409, "Minimum"=w402, "Maximum"=w403, "Increment"=w404) -> ()  [unwired: 2 in, 2 out]
            n295 = property on="V Width" class="DigNum (strict)"("Value"=w410, "Minimum"=w405, "Maximum"=w406, "Increment"=w407) -> ()  [unwired: 2 in, 2 out]
            n296 = local write "SHO"(w398) -> ()
            n297 = local write "SVO"(w408) -> ()
            n298 = local write "SHW"(w409) -> ()
            n299 = local write "SVW"(w410) -> ()
            n300 = call <userlib>:"tm_preparecapture.vi"("error in (no error)"=w390, "Capture mode"=w389, "Handle in"=w381) -> ("error out"=w388:errorcluster, "Buffer Info"=w386:T7, "Handle out"=w387:u32)  [unwired: 5 in, 1 out]
            n301 = call <userlib>:"tm_startcapture_b.vi"("error in (no error)"=w388, "Handle in"=w387) -> ("error out"=w385:errorcluster, "Handle out"=w384:u32)  [unwired: 8 in]
          }
          frame "Readout Mode" {
            w427 = 1 items=["Snap", "Sequence"] ("Capture mode")
            n302 = call <userlib>:"tm_stopcapture.vi"("error in (no error)"=w432, "Handle in"=w417) -> ("error out"=w433:errorcluster, "Handle out"=w434:u32)  [unwired: 8 in]
            n303 = call <userlib>:"tm_unpreparecapture.vi"("error in (no error)"=w433, "Handle in"=w434) -> ("error out"=w418:errorcluster, "Handle out"=w419:u32)  [unwired: 8 in]
            n304 = local read "Camera Readout Mode"() -> (w430:u16)
            n305 = call <userlib>:"tm_setpropertyvalue.vi"("error in (no error)"=w418, "Value in"=w430, "Property ID"=u32 4194832, "Handle in"=w419) -> ("error out"=w428:errorcluster, "Handle out"=w429:u32)  [unwired: 6 in]
            n306 = case shown="12" w430 {
              tunnel: [w438 w443] -> w421
              tunnel: w429 -> [w437 w444]
              tunnel: w428 -> [w436 w443]
              tunnel: [w435 w442] -> w420
              frame 1, Default {
                n307 = local read "Exposure"() -> (w439:dbl)
                n308 = call <userlib>:"tm_setpropertyvalue.vi"("error in (no error)"=w436, "Value in"=w439, "Property ID"=u32 2031888, "Handle in"=w437) -> ("error out"=w438:errorcluster, "Handle out"=w435:u32)  [unwired: 6 in]
              }
              frame 12 {
                n309 = local read "Slit Width / Lines"() -> (w441:sgl)
                n310 = local read "Exposure"() -> (w451:dbl)
                n311 = local read "SVW"() -> (w450:i32)
                n312 = formula code="slitExpos=frameInter*LW/(LinesToReadout\n+10+LW);\nlineInter = slitExpos / LW;"("frameInter"=w451, "LW"=w441, "LinesToReadout"=w450) -> ("slitExpos"=w445:dbl, "lineInter"=w448:dbl)
                n313 = call <userlib>:"tm_setpropertyvalue.vi"("Value in"=w448, "Property ID"=u32 4208720, "Handle in"=w444) -> ("Handle out"=w447:u32)  [unwired: 7 in, 1 out]
                n314 = call <userlib>:"tm_setpropertyvalue.vi"("Value in"=w445, "Property ID"=u32 2031888, "Handle in"=w447) -> ("Handle out"=w442:u32)  [unwired: 7 in, 1 out]
              }
            }
            n315 = call <userlib>:"tm_preparecapture.vi"("error in (no error)"=w421, "Capture mode"=w427, "Handle in"=w420) -> ("error out"=w426:errorcluster, "Buffer Info"=w424:T7, "Handle out"=w425:u32)  [unwired: 5 in, 1 out]
            n316 = call <userlib>:"tm_startcapture_b.vi"("error in (no error)"=w426, "Handle in"=w425) -> ("error out"=w423:errorcluster, "Handle out"=w422:u32)  [unwired: 8 in]
          }
          frame "Update" {
            w459 = u32 1066144 items=["SENSOR MODE"=4212128, "CCD MODE"=4212384, "READOUT MODE"=4211872, "ACTIVE VIEW INDEX"=4343136, "BITS PER CHANNEL"=4342976, "IMAGE PIXEL TYPE"=4343296, "BINNING"=4215968, "EXPOSURE TIME"=2049184, "CONTRAST GAIN"=3163312, "CONTRAST OFFSET"=3163328, "LIGHT MODE"=2114720, "SENSITIVITY"=2114992, "PHOTON IMAGING MODE"=2115200, "HIGH DYNAMIC RANGE MODE"=3163360, "WHITE BALANCE"=3163568, "TEMPERATURE"=2115232, "TEMPERATURE TARGET"=2115264, "SENSOR COOLER FAN"=2115296, "LINEBUNDLE HEIGHT"=4212192, "MECHANICAL SHUTTER"=2115488, "BACK FOCUS POSITION"=8422304, "TRIGGER CONNECTOR"=1066432, "TRIGGER SOURCE"=1066144, "OUTPUT TRIGGER SOURCE"=1852576, "TRIGGER GLOBAL EXPOSURE"=2049680, "FIRST TRIGGER BEHAVIOR"=2049696, "CHANNEL SYNC"=1852352, "READOUT DIRECTION"=4211904, "PRE HSYNC COUNT"=1852704] ("Parameter")
            w464 = u32 2049184 items=["SENSOR MODE"=4212128, "CCD MODE"=4212384, "READOUT MODE"=4211872, "ACTIVE VIEW INDEX"=4343136, "BITS PER CHANNEL"=4342976, "IMAGE PIXEL TYPE"=4343296, "BINNING"=4215968, "EXPOSURE TIME"=2049184, "CONTRAST GAIN"=3163312, "CONTRAST OFFSET"=3163328, "LIGHT MODE"=2114720, "SENSITIVITY"=2114992, "PHOTON IMAGING MODE"=2115200, "HIGH DYNAMIC RANGE MODE"=3163360, "WHITE BALANCE"=3163568, "TEMPERATURE"=2115232, "TEMPERATURE TARGET"=2115264, "SENSOR COOLER FAN"=2115296, "LINEBUNDLE HEIGHT"=4212192, "MECHANICAL SHUTTER"=2115488, "BACK FOCUS POSITION"=8422304, "TRIGGER CONNECTOR"=1066432, "TRIGGER SOURCE"=1066144, "OUTPUT TRIGGER SOURCE"=1852576, "TRIGGER GLOBAL EXPOSURE"=2049680, "FIRST TRIGGER BEHAVIOR"=2049696, "CHANNEL SYNC"=1852352, "READOUT DIRECTION"=4211904, "PRE HSYNC COUNT"=1852704] ("Parameter")
            # "Fails"
            # "Error on get"
            n317 = local read "Exposure"() -> (w466:dbl)
            n318 = disable-structure shown="Disabled" {
              disable-tunnel: w455 -> [w471 _]
              disable-tunnel: w454 -> [w470 _]
              frame Disabled {
                w469 = u32 4226016 items=["SENSOR MODE"=4212128, "CCD MODE"=4212384, "READOUT MODE"=4211872, "ACTIVE VIEW INDEX"=4343136, "BITS PER CHANNEL"=4342976, "IMAGE PIXEL TYPE"=4343296, "BINNING"=4215968, "EXPOSURE TIME"=2049184, "CONTRAST GAIN"=3163312, "CONTRAST OFFSET"=3163328, "LIGHT MODE"=2114720, "SENSITIVITY"=2114992, "PHOTON IMAGING MODE"=2115200, "HIGH DYNAMIC RANGE MODE"=3163360, "WHITE BALANCE"=3163568, "TEMPERATURE"=2115232, "TEMPERATURE TARGET"=2115264, "SENSOR COOLER FAN"=2115296, "LINEBUNDLE HEIGHT"=4212192, "MECHANICAL SHUTTER"=2115488, "BACK FOCUS POSITION"=8422304, "TRIGGER CONNECTOR"=1066432, "TRIGGER SOURCE"=1066144, "OUTPUT TRIGGER SOURCE"=1852576, "TRIGGER GLOBAL EXPOSURE"=2049680, "FIRST TRIGGER BEHAVIOR"=2049696, "CHANNEL SYNC"=1852352, "READOUT DIRECTION"=4211904, "PRE HSYNC COUNT"=1852704, "INTERNAL LINE SPEED"=4226000, "INTERNAL LINE INTERVAL"=4226016] ("Parameter")
                n319 = local read "Internal Line Interval"() -> (w473:dbl)
                n320 = call <userlib>:"tm_setparameter_a.vi"("error in (no error)"=w470, "Value in"=w473, "Parameter"=w469, "Handle in"=w471) -> ("error out"=w472:errorcluster, "Handle out"=w475:u32)  [unwired: 6 in]
                n321 = call <userlib>:"tm_getparameter_a.vi"("error in (no error)"=w472, "Parameter"=w469, "Handle in"=w475) -> ("Value out"=w474:dbl)  [unwired: 6 in, 2 out]
                n322 = local write "Internal Line Interval"(w474) -> ()
              }
              frame Enabled {
              }
            }
            n323 = call <userlib>:"tm_setparameter_a.vi"("error in (no error)"=w454, "Value in"=w466, "Parameter"=w464, "Handle in"=w455) -> ("error out"=w468:errorcluster, "Handle out"=w465:u32)  [unwired: 6 in]
            n324 = call <userlib>:"tm_getparameter_a.vi"("error in (no error)"=w468, "Parameter"=w464, "Handle in"=w465) -> ("Value out"=w467:dbl)  [unwired: 6 in, 2 out]
            n325 = local write "EXP"(w467) -> ()
            n326 = local read "Trigger Source"() -> (w457:sgl)
            n327 = call <userlib>:"tm_setparameter_a.vi"("error in (no error)"=w454, "Value in"=w457, "Parameter"=w459, "Handle in"=w455) -> ("error out"=w456:errorcluster, "Handle out"=w460:u32)  [unwired: 6 in]
            n328 = call <userlib>:"tm_getparameter_a.vi"("error in (no error)"=w456, "Parameter"=w459, "Handle in"=w460) -> ("error out"=w461:errorcluster, "Value out"=w458:dbl, "Handle out"=w463:u32)  [unwired: 6 in]
            n329 = local write "Trigger Source"(w458) -> ()
          }
          frame "Preview", Default {
            # "Slows it all down somewhat"
            # "Currently the external trigger setting means that frames are dropped because the system lingers at this point. \nIdeally I should set it so when the system is external and recording it won't run this section.\n\nThis is what HC Image does, it offers no live video when you switch from live to record mode.\n\nRealistically when tirgger set external and this times out once then ignore this step.\nBut it'd have to be reset after a recording.\n\nNeed to think more betterer about how to handle this else frames will just be dropped. Probably best to just have a seperate scan mode\nOr at least just a boolean to turn off this live capture section. Working now maybe"
            n330 = call <userlib>:"tm_waitnextframe.vi"("error in (no error)"=w481, "Timeout"=3000, "Handle in"=w490) -> ("error out"=w477:errorcluster, "Handle out"=w478:u32)  [unwired: 5 in, 2 out]
            n331 = call <userlib>:"tm_getframe_a.vi"("error in (no error)"=w477, "Buffer Info"=w484, "Handle in"=w478) -> ("error out"=w482:errorcluster, "Data 16"=w480:u16[][], "Handle out"=w483:u32)  [unwired: 4 in, 2 out]
            n332 = Bundle By Name(cluster=w488, "State"=Stack_Track."Idle", "Stack Number"=0, "Image"=w480) -> (w485:T3)
            n333 = Enqueue Element(queue=w489, element=w485) -> ()  [unwired: 2 in, 3 out]
          }
          frame "Idle" {
          }
          frame "Scan Mode" {
            w499 = 1 items=["Snap", "Sequence"] ("Capture mode")
            w508 = u32 4211872 items=["SENSOR MODE"=4212128, "CCD MODE"=4212384, "READOUT MODE"=4211872, "ACTIVE VIEW INDEX"=4343136, "BITS PER CHANNEL"=4342976, "IMAGE PIXEL TYPE"=4343296, "BINNING"=4215968, "EXPOSURE TIME"=2049184, "CONTRAST GAIN"=3163312, "CONTRAST OFFSET"=3163328, "LIGHT MODE"=2114720, "SENSITIVITY"=2114992, "PHOTON IMAGING MODE"=2115200, "HIGH DYNAMIC RANGE MODE"=3163360, "WHITE BALANCE"=3163568, "TEMPERATURE"=2115232, "TEMPERATURE TARGET"=2115264, "SENSOR COOLER FAN"=2115296, "LINEBUNDLE HEIGHT"=4212192, "MECHANICAL SHUTTER"=2115488, "BACK FOCUS POSITION"=8422304, "TRIGGER CONNECTOR"=1066432, "TRIGGER SOURCE"=1066144, "OUTPUT TRIGGER SOURCE"=1852576, "TRIGGER GLOBAL EXPOSURE"=2049680, "FIRST TRIGGER BEHAVIOR"=2049696, "CHANNEL SYNC"=1852352, "READOUT DIRECTION"=4211904, "PRE HSYNC COUNT"=1852704] ("Parameter")
            n334 = call <userlib>:"tm_stopcapture.vi"("error in (no error)"=w515, "Handle in"=w512) -> ("error out"=w514:errorcluster, "Handle out"=w513:u32)  [unwired: 8 in]
            n335 = call <userlib>:"tm_unpreparecapture.vi"("error in (no error)"=w514, "Handle in"=w513) -> ("error out"=w510:errorcluster, "Handle out"=w511:u32)  [unwired: 8 in]
            n336 = local read "Scan Mode"() -> (w509:dbl)
            n337 = call <userlib>:"tm_setparameter_a.vi"("error in (no error)"=w510, "Value in"=w509, "Parameter"=w508, "Handle in"=w511) -> ("error out"=w504:errorcluster)  [unwired: 6 in, 1 out]
            n338 = call <userlib>:"tm_getparameter_a.vi"("error in (no error)"=w504, "Parameter"=w508) -> ("error out"=w505:errorcluster, "Value out"=w507:dbl, "Handle out"=w500:u32)  [unwired: 7 in]
            n339 = local write "SMD"(w507) -> ()
            n340 = call <userlib>:"tm_preparecapture.vi"("error in (no error)"=w505, "Capture mode"=w499, "Handle in"=w500) -> ("error out"=w506:errorcluster, "Buffer Info"=w498:T7, "Handle out"=w501:u32)  [unwired: 5 in, 1 out]
            n341 = call <userlib>:"tm_startcapture_b.vi"("error in (no error)"=w506, "Handle in"=w501) -> ("error out"=w503:errorcluster, "Handle out"=w502:u32)  [unwired: 8 in]
          }
          frame "Trigger Mode" {
            w523 = u32 1049104 ("Property ID")
            n342 = local read "Trigger Mode"() -> (w528:sgl)
            n343 = call <userlib>:"tm_stopcapture.vi"("error in (no error)"=w521, "Handle in"=w522) -> ("error out"=w527:errorcluster, "Handle out"=w535:u32)  [unwired: 8 in]
            n344 = call <userlib>:"tm_unpreparecapture.vi"("error in (no error)"=w527, "Handle in"=w535) -> ("error out"=w525:errorcluster, "Handle out"=w531:u32)  [unwired: 8 in]
            n345 = call <userlib>:"tm_setpropertyvalue.vi"("error in (no error)"=w525, "Value in"=w528, "Property ID"=w523, "Handle in"=w531) -> ("error out"=w524:errorcluster, "Handle out"=w530:u32)  [unwired: 6 in]
            n346 = call <userlib>:"tm_getpropertyvalue.vi"("error in (no error)"=w524, "Property ID"=w523, "Handle in"=w530) -> ("error out"=w532:errorcluster, "Value in"=w529:sgl, "Handle out"=w533:u32)  [unwired: 6 in]
            n347 = local write "Trigger Mode"(w529) -> ()
            n348 = call <userlib>:"tm_preparecapture.vi"("error in (no error)"=w532, "Handle in"=w533) -> ("error out"=w526:errorcluster, "Buffer Info"=w520:T7, "Handle out"=w534:u32)  [unwired: 6 in, 1 out]
            n349 = call <userlib>:"tm_startcapture_b.vi"("error in (no error)"=w526, "Handle in"=w534) -> ("error out"=w518:errorcluster, "Handle out"=w519:u32)  [unwired: 8 in]
          }
          frame "Readout Direction" {
            w536 = u32 4211904 items=["SENSOR MODE"=4212128, "CCD MODE"=4212384, "READOUT MODE"=4211872, "ACTIVE VIEW INDEX"=4343136, "BITS PER CHANNEL"=4342976, "IMAGE PIXEL TYPE"=4343296, "BINNING"=4215968, "EXPOSURE TIME"=2049184, "CONTRAST GAIN"=3163312, "CONTRAST OFFSET"=3163328, "LIGHT MODE"=2114720, "SENSITIVITY"=2114992, "PHOTON IMAGING MODE"=2115200, "HIGH DYNAMIC RANGE MODE"=3163360, "WHITE BALANCE"=3163568, "TEMPERATURE"=2115232, "TEMPERATURE TARGET"=2115264, "SENSOR COOLER FAN"=2115296, "LINEBUNDLE HEIGHT"=4212192, "MECHANICAL SHUTTER"=2115488, "BACK FOCUS POSITION"=8422304, "TRIGGER CONNECTOR"=1066432, "TRIGGER SOURCE"=1066144, "OUTPUT TRIGGER SOURCE"=1852576, "TRIGGER GLOBAL EXPOSURE"=2049680, "FIRST TRIGGER BEHAVIOR"=2049696, "CHANNEL SYNC"=1852352, "READOUT DIRECTION"=4211904, "PRE HSYNC COUNT"=1852704, "INTERNAL LINE SPEED"=4226000, "INTERNAL LINE INTERVAL"=4226016] ("Parameter")
            w547 = 1 items=["Snap", "Sequence"] ("Capture mode")
            n350 = call <userlib>:"tm_stopcapture.vi"("error in (no error)"=w546, "Handle in"=w556) -> ("error out"=w548:errorcluster, "Handle out"=w555:u32)  [unwired: 8 in]
            n351 = call <userlib>:"tm_unpreparecapture.vi"("error in (no error)"=w548, "Handle in"=w555) -> ("error out"=w549:errorcluster, "Handle out"=w554:u32)  [unwired: 8 in]
            n352 = local read "Readout Direction"() -> (w539:sgl)
            n353 = call <userlib>:"tm_setparameter_a.vi"("error in (no error)"=w549, "Value in"=w539, "Parameter"=w536, "Handle in"=w554) -> ("error out"=w543:errorcluster, "Handle out"=w545:u32)  [unwired: 6 in]
            n354 = call <userlib>:"tm_getparameter_a.vi"("error in (no error)"=w543, "Parameter"=w536, "Handle in"=w545) -> ("error out"=w542:errorcluster, "Value out"=w541:dbl, "Handle out"=w544:u32)  [unwired: 6 in]
            n355 = local write "Readout Direction"(w541) -> ()
            n356 = call <userlib>:"tm_preparecapture.vi"("error in (no error)"=w542, "Capture mode"=w547, "Handle in"=w544) -> ("error out"=w550:errorcluster, "Buffer Info"=w540:T7, "Handle out"=w553:u32)  [unwired: 5 in, 1 out]
            n357 = call <userlib>:"tm_startcapture_b.vi"("error in (no error)"=w550, "Handle in"=w553) -> ("error out"=w551:errorcluster, "Handle out"=w552:u32)  [unwired: 8 in]
          }
          frame "IntervalLineInt" {
            w557 = 4226016
            w568 = 1 items=["Snap", "Sequence"] ("Capture mode")
            n358 = call <userlib>:"tm_stopcapture.vi"("error in (no error)"=w567, "Handle in"=w577) -> ("error out"=w569:errorcluster, "Handle out"=w576:u32)  [unwired: 8 in]
            n359 = call <userlib>:"tm_unpreparecapture.vi"("error in (no error)"=w569, "Handle in"=w576) -> ("error out"=w570:errorcluster, "Handle out"=w575:u32)  [unwired: 8 in]
            n360 = local read "Internal Line Interval"() -> (w560:dbl)
            n361 = call <userlib>:"tm_setparameter_a.vi"("error in (no error)"=w570, "Value in"=w560, "Parameter"=w557, "Handle in"=w575) -> ("error out"=w564:errorcluster, "Handle out"=w566:u32)  [unwired: 6 in]
            n362 = call <userlib>:"tm_getparameter_a.vi"("error in (no error)"=w564, "Parameter"=w557, "Handle in"=w566) -> ("error out"=w563:errorcluster, "Value out"=w562:dbl, "Handle out"=w565:u32)  [unwired: 6 in]
            n363 = local write "Internal Line Interval"(w562) -> ()
            n364 = call <userlib>:"tm_preparecapture.vi"("error in (no error)"=w563, "Capture mode"=w568, "Handle in"=w565) -> ("error out"=w571:errorcluster, "Buffer Info"=w561:T7, "Handle out"=w574:u32)  [unwired: 5 in, 1 out]
            n365 = call <userlib>:"tm_startcapture_b.vi"("error in (no error)"=w571, "Handle in"=w574) -> ("error out"=w572:errorcluster, "Handle out"=w573:u32)  [unwired: 8 in]
          }
          frame "Disengage Update" {
          }
        }
        n366 = local read "stop"() -> (w163:bool)
        n367 = Compound Arithmetic op=OR(w163, w162) -> (w161:bool)
      }
      n368 = while {
        tunnel: w14 -> [w1107]
        shift-right: [w1103] -> _
        shift-left: _ -> [w1101]
        shift-right: [w1100] -> _
        shift-left: w9 -> [w1093]
        shift-right: [w1098] -> _
        shift-left: _ -> [w1094]
        stop <- w1102 stop-if-true
        n369 = Dequeue Element(queue=w1107, error in (no error)=w1093) -> (element=w1106:T3, timed out?=w1095:bool, error out=w1092:errorcluster)  [unwired: 1 in, 1 out]
        n370 = Unbundle By Name(w1106) -> ("State"=w1105:T1, "Stack Number"=w1104:i32, "Image"=w1096:u16[][])
        "State" <- w1105
        n371 = case shown="False" w1095 {
          tunnel: w1096 -> [w1109 w1111]
          tunnel: [w1109 w1110] -> w1097
          tunnel: [w1108 w1111] -> w1098
          tunnel: w1094 -> [w1108 w1110]
          frame False {
          }
          frame True {
          }
        }
        "Image" <- w1097
        n372 = case shown="\"Collecting\"" w1105 {
          tunnel: w1104 -> [_ _ _ _ _ _]
          tunnel: [w1114 w1131 _ _ _ _] -> w1103
          tunnel: w1101 -> [_ w1132 w1138 _ _ _]
          tunnel: [FALSE _ _ _ TRUE _] -> w1102
          tunnel: w1097 -> [w1112 w1133 _ _ _ _]
          tunnel: w1092 -> [_ w1130 w1136 w1148 w1173 w1175]
          tunnel: [w1115 w1129 w1137 w1145 w1173 w1175] -> w1100
          tunnel: "Path" -> [w1118 _ _ w1150 _ _]
          frame "Start Sequence" {
            # "Public tiff library"
            # "Get path and open file"
            n373 = Equal?(x=w1118, y=path "") -> (x = y?=w1120:bool)
            n374 = case shown="True" w1120 {
              tunnel: w1118 -> [w1122 _]
              tunnel: [w1122 w1125] -> w1117
              frame False {
              }
              frame True {
                n375 = call "File Dialog"("pattern (all files)"=".tiff", "pattern label"="Tiff Image") -> ("selected path"=w1125:path)  [unwired: 10 in, 3 out]
              }
            }
            n376 = case shown="True" "AutoIncrement" {
              tunnel: w1117 -> [w1126 w1128]
              tunnel: [w1126 w1127] -> w1113
              frame False {
              }
              frame True {
                n377 = call "4Digit File Incrementer.vi"("path"=w1128) -> ("appended path"=w1127:path)  [unwired: 10 in]
              }
            }
            n378 = local write "Path"(w1113) -> ()
            n379 = call-poly "CTIFFNewFileAndStyle.vi"("image"=w1112, "output_file"=w1113) -> ("error"=w1115:errorcluster, "CTIFF"=w1114:i64)  [unwired: 8 in]
          }
          frame "Collecting" {
            # "Add Image to write scan line"
            n380 = call-poly "CTIFFAddNewPage.vi"("error"=w1130, "image"=w1133, "CTIFF"=w1132) -> ("error"=w1129:errorcluster, "CTIFF"=w1131:i64)  [unwired: 7 in]
            n381 = property on="Ram Record" class="Bool (strict)"("DisabledEnum"=T4."Disabled and Grayed Out" ("Disabled"), "BoolText.Text"="Saving" ("Boolean Text.Text")) -> ()  [unwired: 2 in, 2 out]
          }
          frame "End" {
            (unwired) FALSE
            # "Close image file, reset capturing button"
            n382 = call "CTIFFWriteAndClose.vi"("error"=w1136, "CTIFF"=w1138) -> ("error"=w1137:errorcluster)  [unwired: 9 in]
            n383 = property on="Ram Record" class="Bool (strict)"("BoolText.Text"="OK" ("Boolean Text.Text"), "DisabledEnum"=T4."Enabled" ("Disabled")) -> ()  [unwired: 2 in, 2 out]
          }
          frame "Read Disk" {
            w1141 = path "C:/temp.tmp" ("Temp 2")
            # "Can't just send hardisk record in a loop a bunch of times though.\nHave to modify consumer"
            # "This is the easiest option."
            # "Could potentially implments stacks into ram and hardisk record"
            # "For instance the harddisk record may be set to record 5000 images, this could then be used to chunk that into\n50 stacks of 100"
            # "Use stacks one day for rapid imaging , whatevr."
            n384 = call <userlib>:"tm_opendcimgfile.vi"("Path"=w1141) -> ("Total Frames"=w1151:i32, "File Handle"=w1152:u32)  [unwired: 8 in, 1 out]
            n385 = for {
              N: w1151 -> [_]
              tunnel: w1150 -> [w1160]
              shift-right: [w1158] -> w1146
              shift-left: i64 0 ("CTIFF") -> [w1159]
              tunnel: [w1157] -> w1147
              tunnel: w1148 -> [w1156]
              shift-right: [w1162] -> w1142
              shift-left: w1152 -> [w1163]
              i -> [w1153]
              n386 = local write "Stack Frames"(w1153) -> ()
              n387 = Equal To 0?(x=w1153) -> (x = 0?=w1161:bool)
              n388 = call <userlib>:"tm_getdcimgframe.vi"("error in (no error)"=w1156, "Frame Index"=w1153, "File Handle in"=w1163) -> ("error out"=w1155:errorcluster, "Data"=w1154:u16[][], "File Handle out"=w1162:u32)  [unwired: 5 in, 1 out]
              n389 = local write "Image"(w1154) -> ()
              n390 = case shown="True" w1161 {
                tunnel: w1160 -> [_ w1172]
                tunnel: w1154 -> [w1164 w1171]
                tunnel: w1159 -> [w1168 _]
                tunnel: [w1167 w1170] -> w1158
                tunnel: [w1166 w1169] -> w1157
                tunnel: w1155 -> [w1165 _]
                frame False {
                  n391 = call-poly "CTIFFAddNewPage.vi"("error"=w1165, "image"=w1164, "CTIFF"=w1168) -> ("error"=w1166:errorcluster, "CTIFF"=w1167:i64)  [unwired: 7 in]
                }
                frame True {
                  n392 = call-poly "CTIFFNewFileAndStyle.vi"("image"=w1171, "output_file"=w1172) -> ("error"=w1169:errorcluster, "CTIFF"=w1170:i64)  [unwired: 8 in]
                }
              }
            }
            n393 = call "CTIFFWriteAndClose.vi"("error"=w1147, "CTIFF"=w1146) -> ("error"=w1144:errorcluster)  [unwired: 9 in]
            n394 = call <userlib>:"tm_closedcimgfile.vi"("error in (no error)"=w1144, "File Handle"=w1142) -> ("error out"=w1143:errorcluster)  [unwired: 9 in]
            n395 = Delete(path (use dialog)=w1141, error in=w1143) -> (error out=w1145:errorcluster)  [unwired: 3 in, 2 out]
          }
          frame "STOP" {
          }
          frame "Idle" {
          }
        }
      }
      n396 = while {
        tunnel: w17 -> [w100]
        stop <- "stop" stop-if-true
        n397 = event shown="[13] \"Internal Line Interval\": Value Change" {
          selector: _ -> [_ _ _ _ _ _ _ _ _ _ _ _ _ _]
          dyn-events: _ -> [_ _ _ _ _ _ _ _ _ _ _ _ _ _]
          timeout: _ -> [_ _ _ _ _ _ _ _ _ _ _ _ _ _]
          tunnel: w100 -> [_ w102 w104 w105 w107 w110 w113 w117 w123 w129 w132 w136 w146 w156]
          event Timeout {
            n398 = event-data() -> ()  [unwired: 1 in, 3 out]
          }
          event "Camera Readout Mode": Value Change {
            n399 = event-data() -> ()  [unwired: 1 in, 6 out]
            n400 = Enqueue Element(queue=w102, element=CameraControlTypeDef."Readout Mode" ("Enum")) -> ()  [unwired: 2 in, 3 out]
          }
          event "V Width", "V Offset", "H Width", "H Offset": Value Change {
            n401 = event-data() -> ()  [unwired: 1 in, 6 out]
            n402 = Enqueue Element(queue=w104, element=CameraControlTypeDef."ROI" ("Enum")) -> ()  [unwired: 2 in, 3 out]
          }
          event "Readout Direction": Value Change {
            n403 = event-data() -> ()  [unwired: 1 in, 6 out]
            n404 = Enqueue Element(queue=w105, element=CameraControlTypeDef."Readout Direction" ("Enum")) -> ()  [unwired: 2 in, 3 out]
          }
          event "Binning": Value Change {
            n405 = event-data() -> ()  [unwired: 1 in, 6 out]
            n406 = Enqueue Element(queue=w107, element=CameraControlTypeDef."Binning" ("Enum")) -> ()  [unwired: 2 in, 3 out]
          }
          event "Ram Record": Value Change {
            n407 = event-data() -> ("NewVal"=w109:bool)  [unwired: 1 in, 5 out]
            n408 = case shown="True" w109 {
              tunnel: w110 -> [_ w111]
              frame False {
              }
              frame True {
                n409 = Enqueue Element(queue=w111, element=CameraControlTypeDef."Ram Record" ("Enum")) -> ()  [unwired: 2 in, 3 out]
              }
            }
          }
          event "Capture Mode": Value Change {
            n410 = event-data() -> ("NewVal"=w114:bool)  [unwired: 1 in, 5 out]
            n411 = case shown="True" w114 {
              tunnel: w113 -> [_ w116]
              frame False {
              }
              frame True {
                n412 = Enqueue Element(queue=w116, element=CameraControlTypeDef."Idle") -> ()  [unwired: 2 in, 3 out]
              }
            }
          }
          event "Preview": Value Change {
            n413 = event-data() -> ("NewVal"=w118:bool)  [unwired: 1 in, 5 out]
            n414 = case shown="True" w118 {
              tunnel: w117 -> [_ w120]
              frame False {
              }
              frame True {
                n415 = Enqueue Element(queue=w120, element=CameraControlTypeDef."Preview") -> ()  [unwired: 2 in, 3 out]
              }
            }
          }
          event "Time Lapse": Value Change {
            n416 = event-data() -> ("NewVal"=w122:bool)  [unwired: 1 in, 5 out]
            n417 = for {
              N: "Stacks" -> [_]
              tunnel: w123 -> [w125]
              tunnel: w122 -> [w124]
              n418 = case shown="True" w124 {
                tunnel: w125 -> [_ w127]
                frame False {
                }
                frame True {
                  n419 = Enqueue Element(queue=w127, element=CameraControlTypeDef."Ram Record" ("Enum")) -> ()  [unwired: 2 in, 3 out]
                }
              }
            }
          }
          event "HardDisk Record": Value Change {
            n420 = event-data() -> ("NewVal"=w128:bool)  [unwired: 1 in, 5 out]
            n421 = case shown="True" w128 {
              tunnel: w129 -> [_ w130]
              frame False {
              }
              frame True {
                n422 = Enqueue Element(queue=w130, element=CameraControlTypeDef."HardDisk Record" ("Enum")) -> ()  [unwired: 2 in, 3 out]
              }
            }
          }
          event "Exposure": Value Change {
            n423 = event-data() -> ()  [unwired: 1 in, 6 out]
            n424 = Enqueue Element(queue=w132, element=CameraControlTypeDef."Update" ("Enum")) -> ()  [unwired: 2 in, 3 out]
          }
          event "Trigger Source": Value Change {
            n425 = event-data() -> ("NewVal"=w134:sgl)  [unwired: 1 in, 5 out]
            n426 = case shown="1, Default" w134 {
              tunnel: w136 -> [w139 w142]
              tunnel: [w138 w141] -> w135
              frame 2 {
                n427 = Enqueue Element(queue=w139, element=CameraControlTypeDef."Idle" ("Enum")) -> (queue out=w138:refnum<queue>)  [unwired: 2 in, 2 out]
              }
              frame 1, Default {
                n428 = Enqueue Element(queue=w142, element=CameraControlTypeDef."Preview" ("Enum")) -> (queue out=w141:refnum<queue>)  [unwired: 2 in, 2 out]
              }
            }
            n429 = Enqueue Element(queue=w135, element=CameraControlTypeDef."Update" ("Enum")) -> ()  [unwired: 2 in, 3 out]
          }
          event "Trigger Mode": Value Change {
            n430 = event-data() -> ("NewVal"=w144:sgl)  [unwired: 1 in, 5 out]
            n431 = case shown="6" w144 {
              tunnel: w146 -> [w149 w152]
              tunnel: [w148 w151] -> w145
              frame 6 {
                n432 = Enqueue Element(queue=w149, element=CameraControlTypeDef."Idle" ("Enum")) -> (queue out=w148:refnum<queue>)  [unwired: 2 in, 2 out]
              }
              frame 1, Default {
                n433 = Enqueue Element(queue=w152, element=CameraControlTypeDef."Preview" ("Enum")) -> (queue out=w151:refnum<queue>)  [unwired: 2 in, 2 out]
              }
            }
            n434 = Enqueue Element(queue=w145, element=CameraControlTypeDef."Trigger Mode" ("Enum")) -> ()  [unwired: 2 in, 3 out]
          }
          event "Internal Line Interval": Value Change {
            n435 = event-data() -> ("OldVal"=w155:dbl)  [unwired: 1 in, 5 out]
            n436 = Enqueue Element(queue=w156, element=CameraControlTypeDef."IntervalLineInt", timeout in ms (-1)=w155) -> ()  [unwired: 1 in, 3 out]
          }
        }
      }
      n437 = call <userlib>:"tm_stopcapture.vi"("error in (no error)"=w22, "Handle in"=w23) -> ("error out"=w69:errorcluster, "Handle out"=w70:u32)  [unwired: 8 in]
      n438 = call <userlib>:"tm_unpreparecapture.vi"("error in (no error)"=w69, "Handle in"=w70) -> ("error out"=w68:errorcluster, "Handle out"=w71:u32)  [unwired: 8 in]
      n439 = call <userlib>:"tm_closecamera.vi"("error in (no error)"=w68, "Handle in"=w71) -> ("error out"=w96:errorcluster)  [unwired: 9 in]
      n440 = call <userlib>:"tm_deinitialize.vi"("error in (no error)"=w96) -> ("error out"=w18:errorcluster)  [unwired: 10 in]
      n441 = Release Queue(queue=w17, error in (no error)=w18) -> (error out=w16:errorcluster)  [unwired: 1 in, 2 out]
      n442 = Release Queue(queue=w14, error in (no error)=w16) -> (error out=w15:errorcluster)  [unwired: 1 in, 2 out]
    }
  }
  "error out" <- w3
